vi "hostCommander_dualVStim.vi"() -> ()   [LabVIEW 2014]
uses:
  <vilib>/Platform/TimedLoop/XDataNode/timing_clust.ctl
  <vilib>/Platform/TimedLoop/XDataNode/nitl_modes.ctl
  <vilib>/Platform/TimedLoop/XDataNode/wakeup.ctl
  <vilib>/dex/Stream Element Allocation Mode.ctl
  <vilib>/platform/TimedLoop/XDataNode/XDataNode.xnode
  <resource>/objmgr/ni.dex.rc
  <vilib>/Platform/TimedLoop/XDataNode/XDNodeRunTimeDep.lvlib
  <vilib>/Analysis/NI_AALBase.lvlib
  <vilib>/Analysis/1siggen.llb/Riffle Array (I32).vi
panel:
  in  "allowCorrection 2":bool
  out "Tab Control":enum32{"Host Commander"}(tab)
  out "rightReward":dbl format="%.2f"
  out "leftReward":dbl format="%.2f"
  out "rightLick":dbl format="%.2f"
  out "leftLick":dbl format="%.2f"
  out "reward#":i32=500
  in  "tickRate":u32=1
  in  "displayLength":dbl=10.0
  out "CurTrial#":u16
  out "Digital Waveform Graph":digitalwaveform(graph)
  out "stateMissed":bool
  out "VSmissed":bool
  out "VSbusy":bool=TRUE caption="VS"
  out "stateBusy":bool=TRUE caption="State"
  in  "FileName":string="debug"
  in  "Save data":bool=TRUE
  in  "Tab Control _2":T1(tab)
  in  "trialKey":i32[](array[numeric])
  in  "left":dbl=0.5 format="%.2f"
  in  "right":dbl=0.5 format="%.2f"
  in  "Initializeation Screen":dbl
  in  "Repeat":dbl
  in  "Interleave":bool
  in  "Randominze":bool
  in  "Blank":bool
  in  "Timing":sgl[](array[numeric])=[0.1, 0.2, 0.4, 0.6, 0.8, 1.0]
  in  "Orientation":sgl[](array[numeric])=[0.1, 0.2, 0.4, 0.6, 0.8, 1.0]
  in  "TF":sgl[](array[numeric])=[0.1, 0.2, 0.4, 0.6, 0.8, 1.0]
  in  "VS type":string="LR_FullFiledGrating"
  in  "SF":sgl[](array[numeric])=[0.04, 0.08, 0.16, 0.32, 0.45]
  in  "rtFIFOsize":u32=50
  in  "rtFIFOtimeout":u32
  in  "rtFIFOdataPool":u32=20
  in  "stateMachineCycle_uS":i64=500
  in  "minDelay":i32
  in  "maxDelay":i32=2000000
  in  "autoAllowCorrection":bool
  in  "allowCorrection":bool=TRUE
  in  "autoDelay":bool
  in  "vsFilterPeriod_uS":i32=500 format="%#1.6f"
  in  "lickThreshold_V":fxp<+/-,16,5>=1.0 format="%#.4f"
  in  "vsThreshold_V":fxp<+/-,16,5>=2.0 format="%#.4f"
  in  "audioThreshold_V":fxp<+/-,16,5>=2.2998046875 format="%.4f"
  in  "audioFilterPeriod_uS":i32=500 format="%#1.6f"
  in  "audioOffState_V":fxp<+/-,16,5> format="%#.4f"
  in  "manualShock":bool
  in  "manualWaterRight":bool
  in  "manualWaterLeft":bool
  in  "lickReward":bool
  in  "allowPunish":bool
  in  "beh type":string="LeftRight"
  in  "toneReward":bool
  in  "rwdrefPeriod_uS":u32=1000000
  in  "rewardPeriod_uS":u32=3000000
  in  "waterOn_uS":u32=35000
  in  "timeout_uS":u32
  in  "shockOn_uS":u32
  in  "delay_uS":u32
  out "current state":u16(ring) items=["idle", "vs before", "vs", "vs after", "delay", "tone before", "tone", "tone after", "cycle end", "reward", "reward refractory", "punish", "punish refractory", "timeout", "exit"]
  out "case2":i32
  out "case1":i32
  in  "forceLeftTrial":bool
  in  "forceRightTrial":bool
  in  "forceCorrTrial":bool
  in  "autoCorrTrial":bool
  in  "autoTimeout":bool
  in  "autoStop":bool
  in  "autoStopAtReward#":i32=250
  in  "updateEveryTrial#":u16=10
  in  "maxTimeout":i32=8000000
  out "newStartTrial#":i32
  out "newStartReward#":i32
  out "contNoRewardAccum":i32
  out "contNoReward":i32
  out "contReward":i32
  out "curPerformance":dbl format="%.2f"
  out "overallPerformance":dbl format="%.2f"
  in  "waterPunish":bool
  in  "No VS":bool
  out "Error 1":string
  out "Error 2":string
  out "Originating IP":string="192.168.137.2"
  out "Incoming data":string="TrlDone 1.000 "
  out "stream counter":u32
  out "Is Connected":bool
  out "Available Elements for Writing":i32
  in  "stream writer buffer size":i32=500
  in  "IP_VS":string="192.168.137.3"
  in  "IP_RT":string="192.168.137.2"
  in  "port_remote":u16=9091
  in  "IP_host":string="192.168.137.1"
  in  "port_local":u16=9090
  in  "IP_broadcast":string="192.168.137.255"
  out "INFO":string="Stop 1.000 "
  out "stop - local":bool=TRUE
  in  "Notes":string="14-4"
  in  "Abort":bool caption="run-stop"
  in  "run-stop":bool
  out "dispTimeout":bool
  out "saveTimeout":bool
  out "CurTrial# (remote)":u16
  in  "totalTrial#":u16=600
  out "CurTime":i32
  in  "ITI_ms":dbl=2000.0
  out "CurTime (sec)":i32
  in  "FilePath":string="D:\\BehData\\"
  # "busy"
  # "missed"
  # "min"
  # "sec"
  # "trialProbability"
  # "Errors for debugging"
types:
  T1 = enum32{"Visual Stimuli", "State Machine", "Behavior", "Network", "Notes"}
  T2 = enum16{"open", "replace", "create", "open or create", "replace or create", "replace or create with confirmation"}
  T3 = enum16{"big-endian, network order", "native, host order", "little-endian"}
  T4 = typedef "XDNodeRunTimeDep.lvlib/timing_clust.ctl" = cluster{"Expected End [f-1]":u64, "Actual End [f-1]":u64, "Finished Late? [f-1]":bool, "Expected End [i-1]":u64, "Actual End [i-1]":u64, "Finished Late? [i-1]":bool, "Expected Start [i]":u64, "Actual Start [i]":u64, "Expected Start [f]":u64, "Actual Start [f]":u64, "Source Name":string, "Structure Name":string, "Period":i64, "Deadline":i64, "Offset":i64, "Start":i64, "Priority":i32, "Timeout":i32, "Mode":T5, "Wakeup Reason":T6, "Error":errorcluster, "Source Type":string, "Secondary Source Type":string, "Global End Time":u64, "Global Start Time":u64, "Frame Duration":u64, "Iteration Duration":u64, "Assigned CPU":i32, "I/O Scan Engine Mode":u32}
  T5 = typedef "XDNodeRunTimeDep.lvlib/nitl_modes.ctl" = enum32{"No Change", "Process missed periods, maintain original phase", "Discard missed periods, maintain original phase", "Process missed periods, ignore original phase", "Discard missed periods, ignore original phase"}
  T6 = typedef "XDNodeRunTimeDep.lvlib/wakeup.ctl" = enum32{"Normal", "Aborted", "Asynchronous wakeup", "Timing source error", "Timed loop error", "Timeout"}
  T7 = typedef "Stream Element Allocation Mode.ctl" = u32
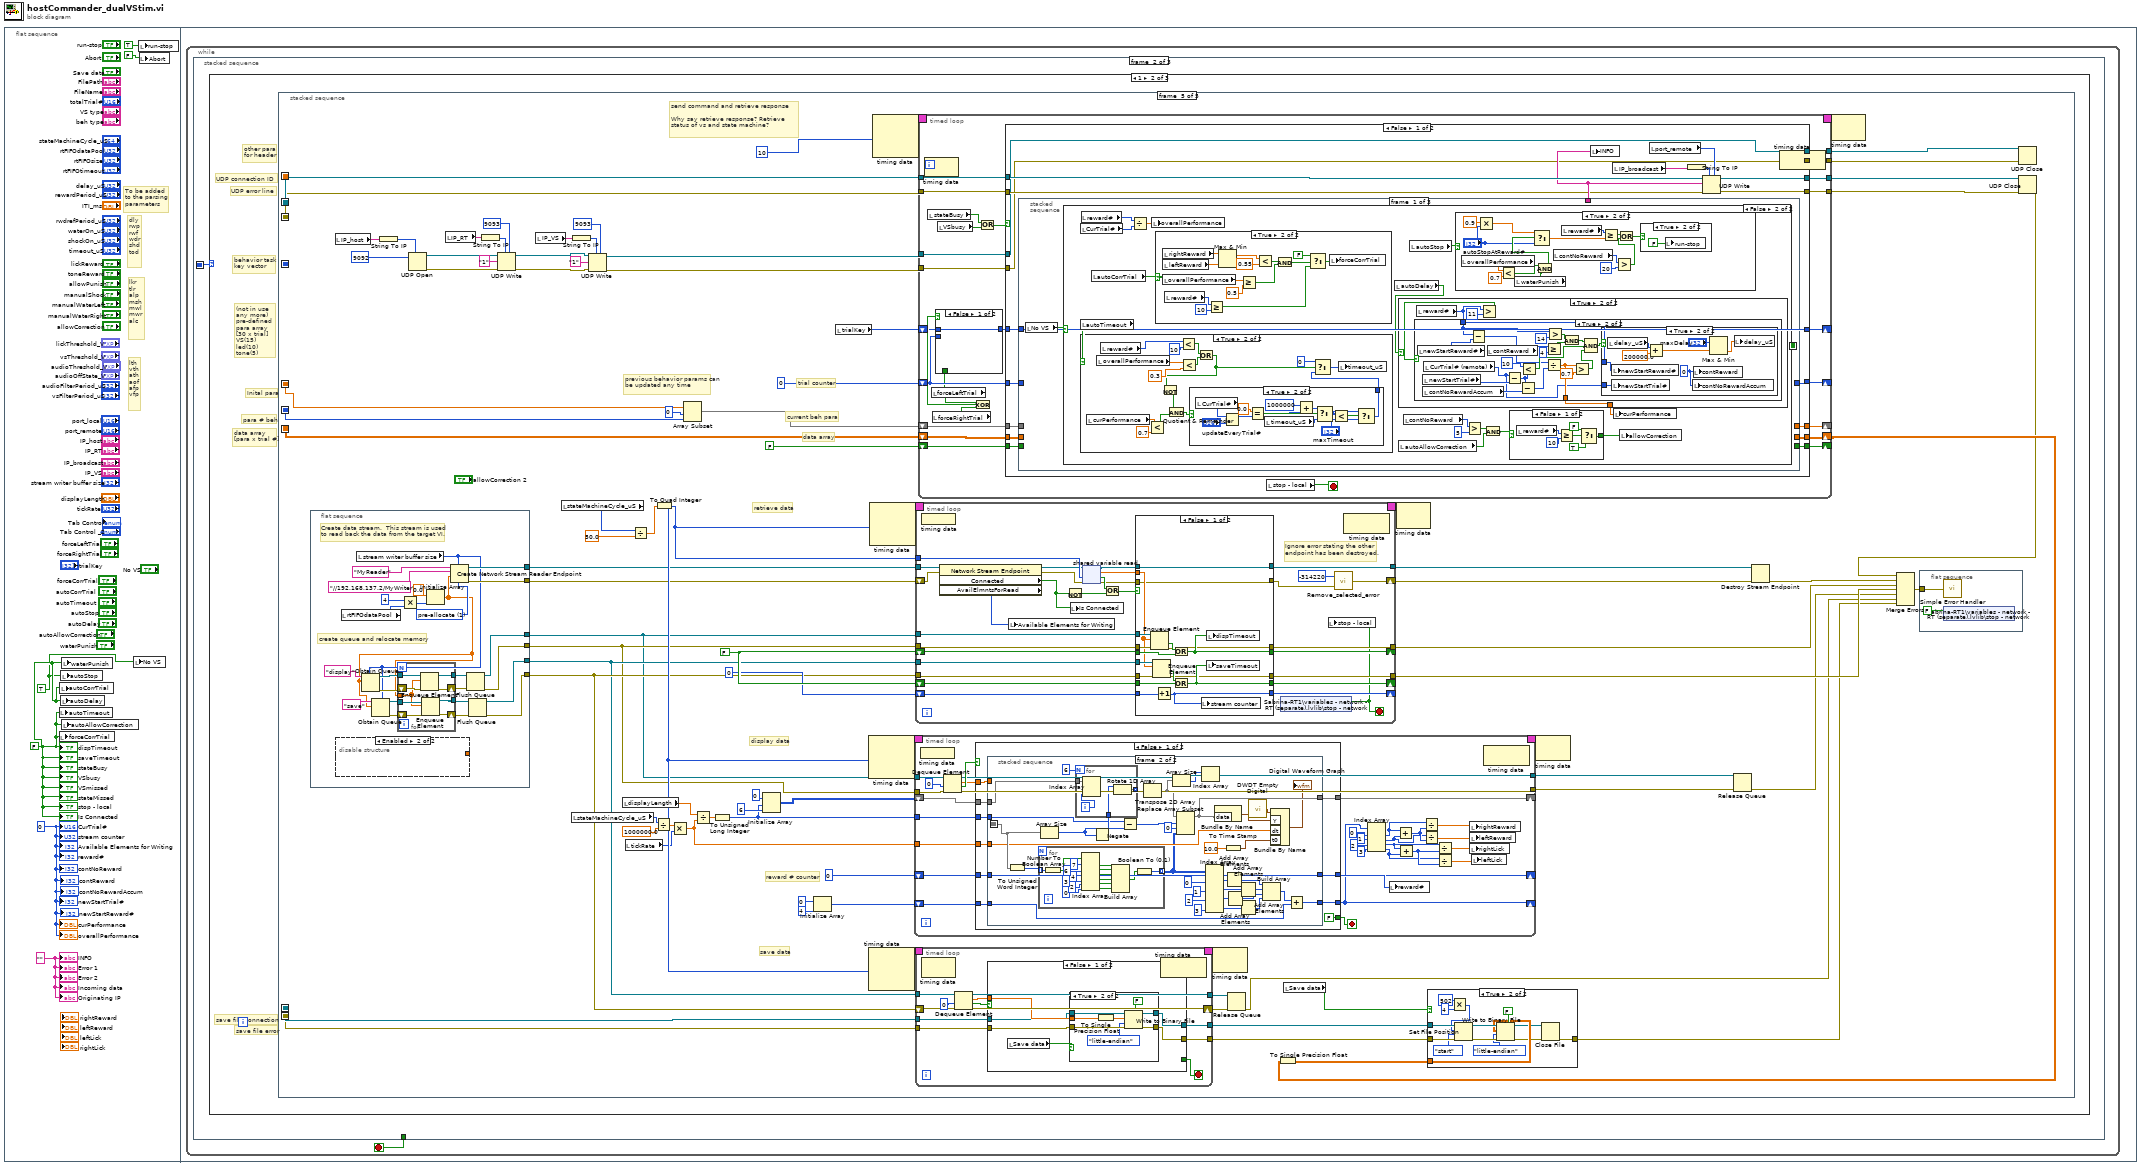
[diagram p0: block diagram]
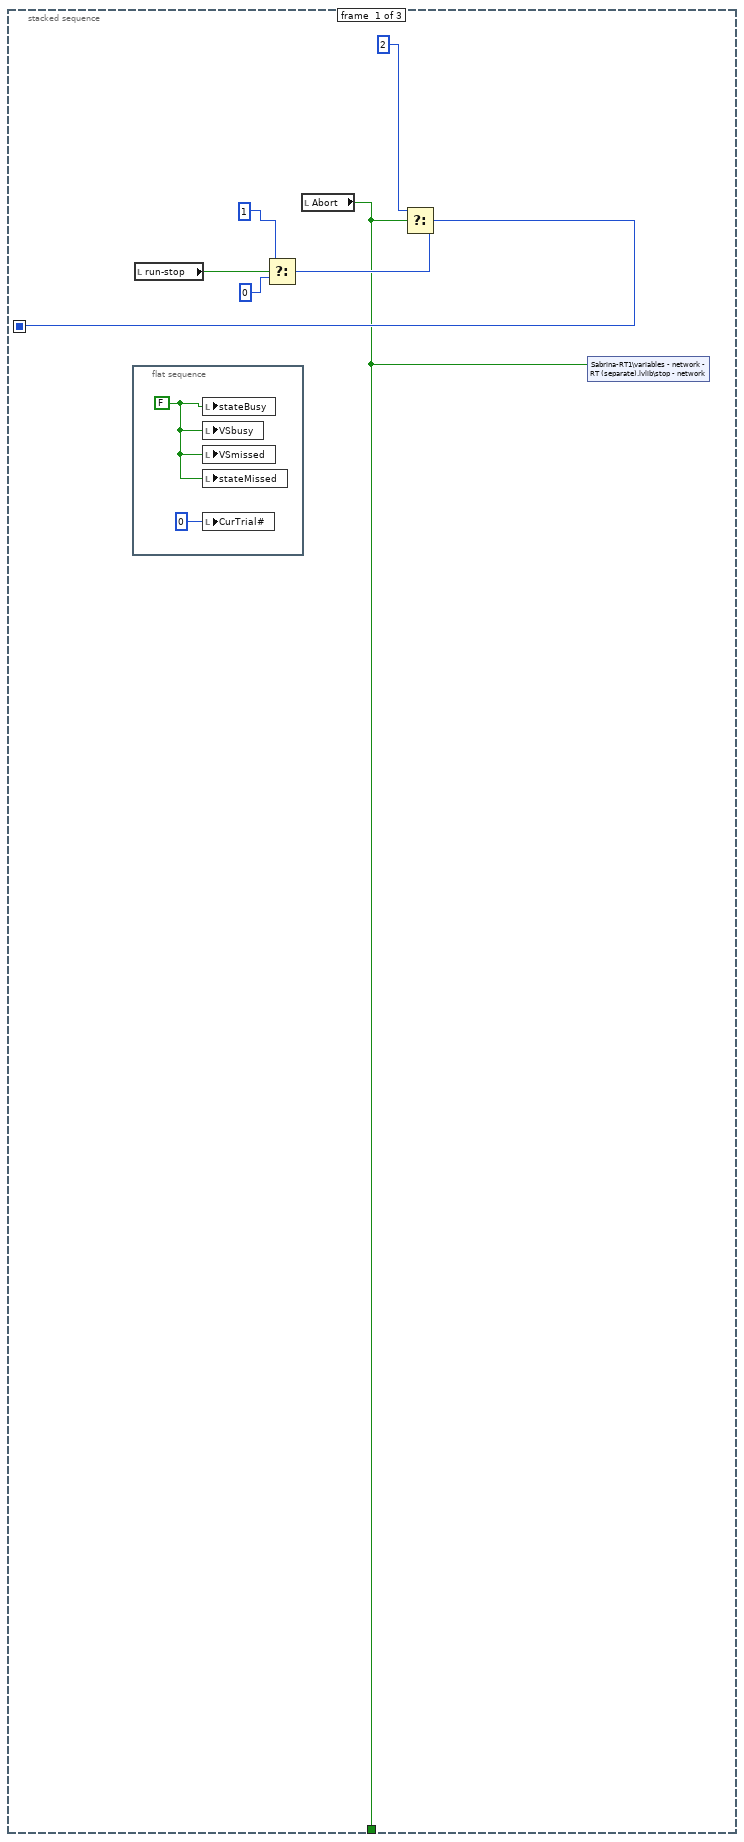
[diagram p2: hidden frame]
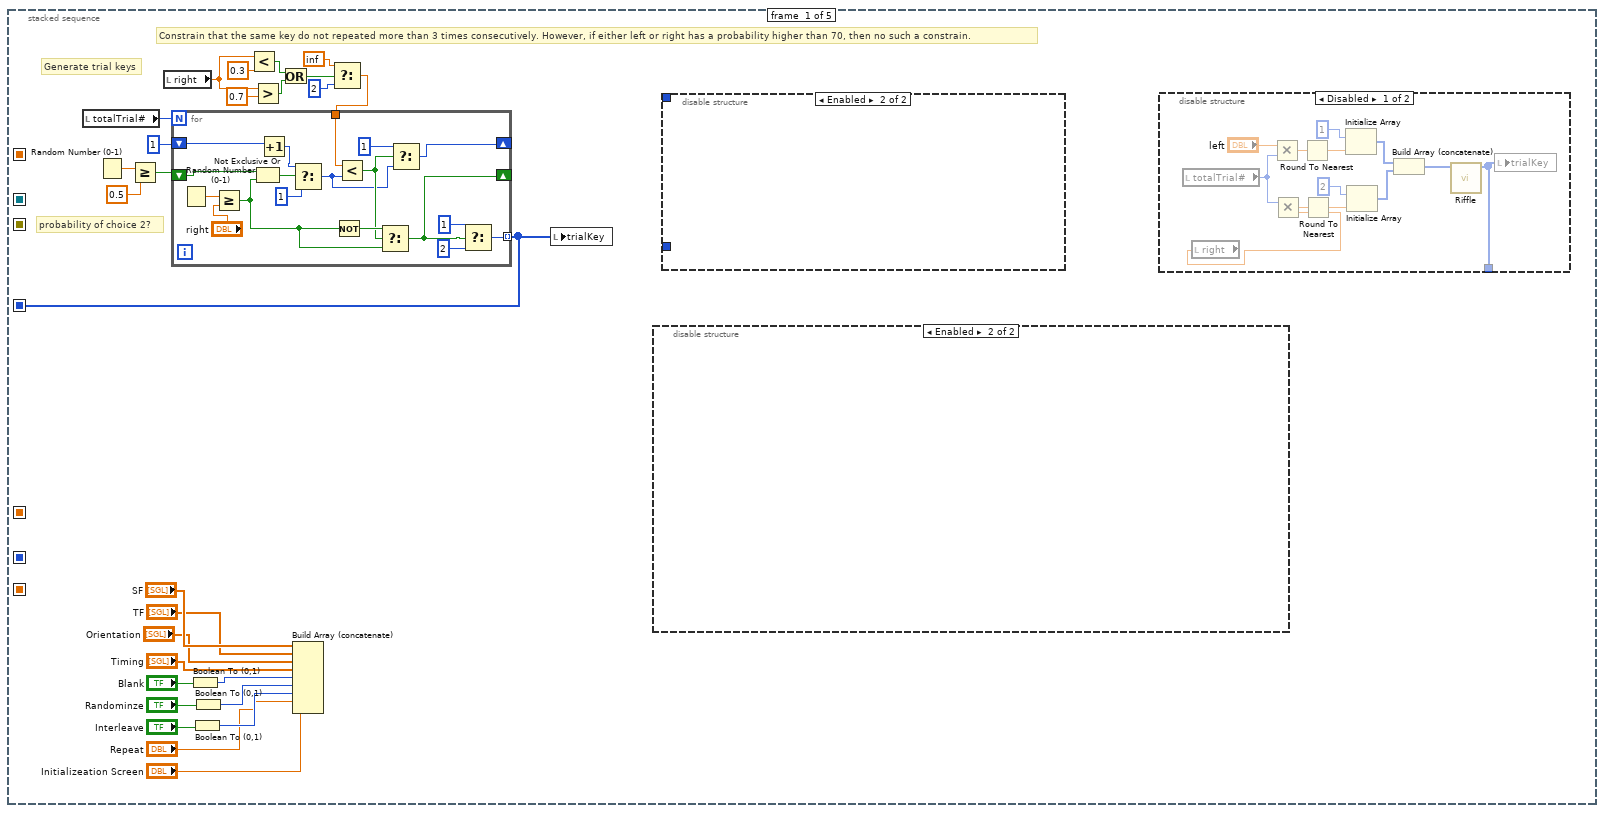
[diagram p4: hidden frame]
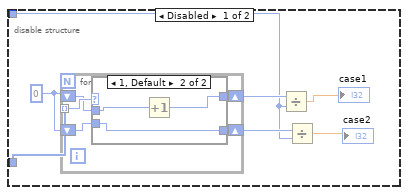
[diagram p5: hidden frame]
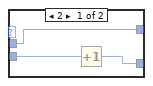
[diagram p6: hidden frame]
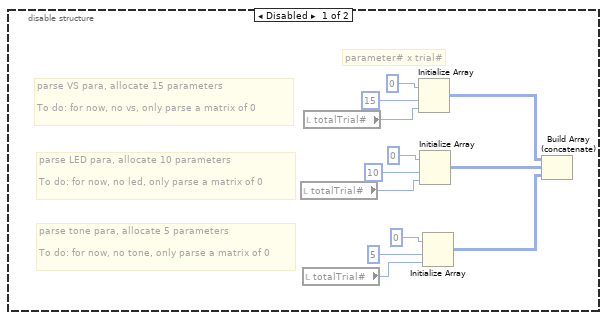
[diagram p8: hidden frame]
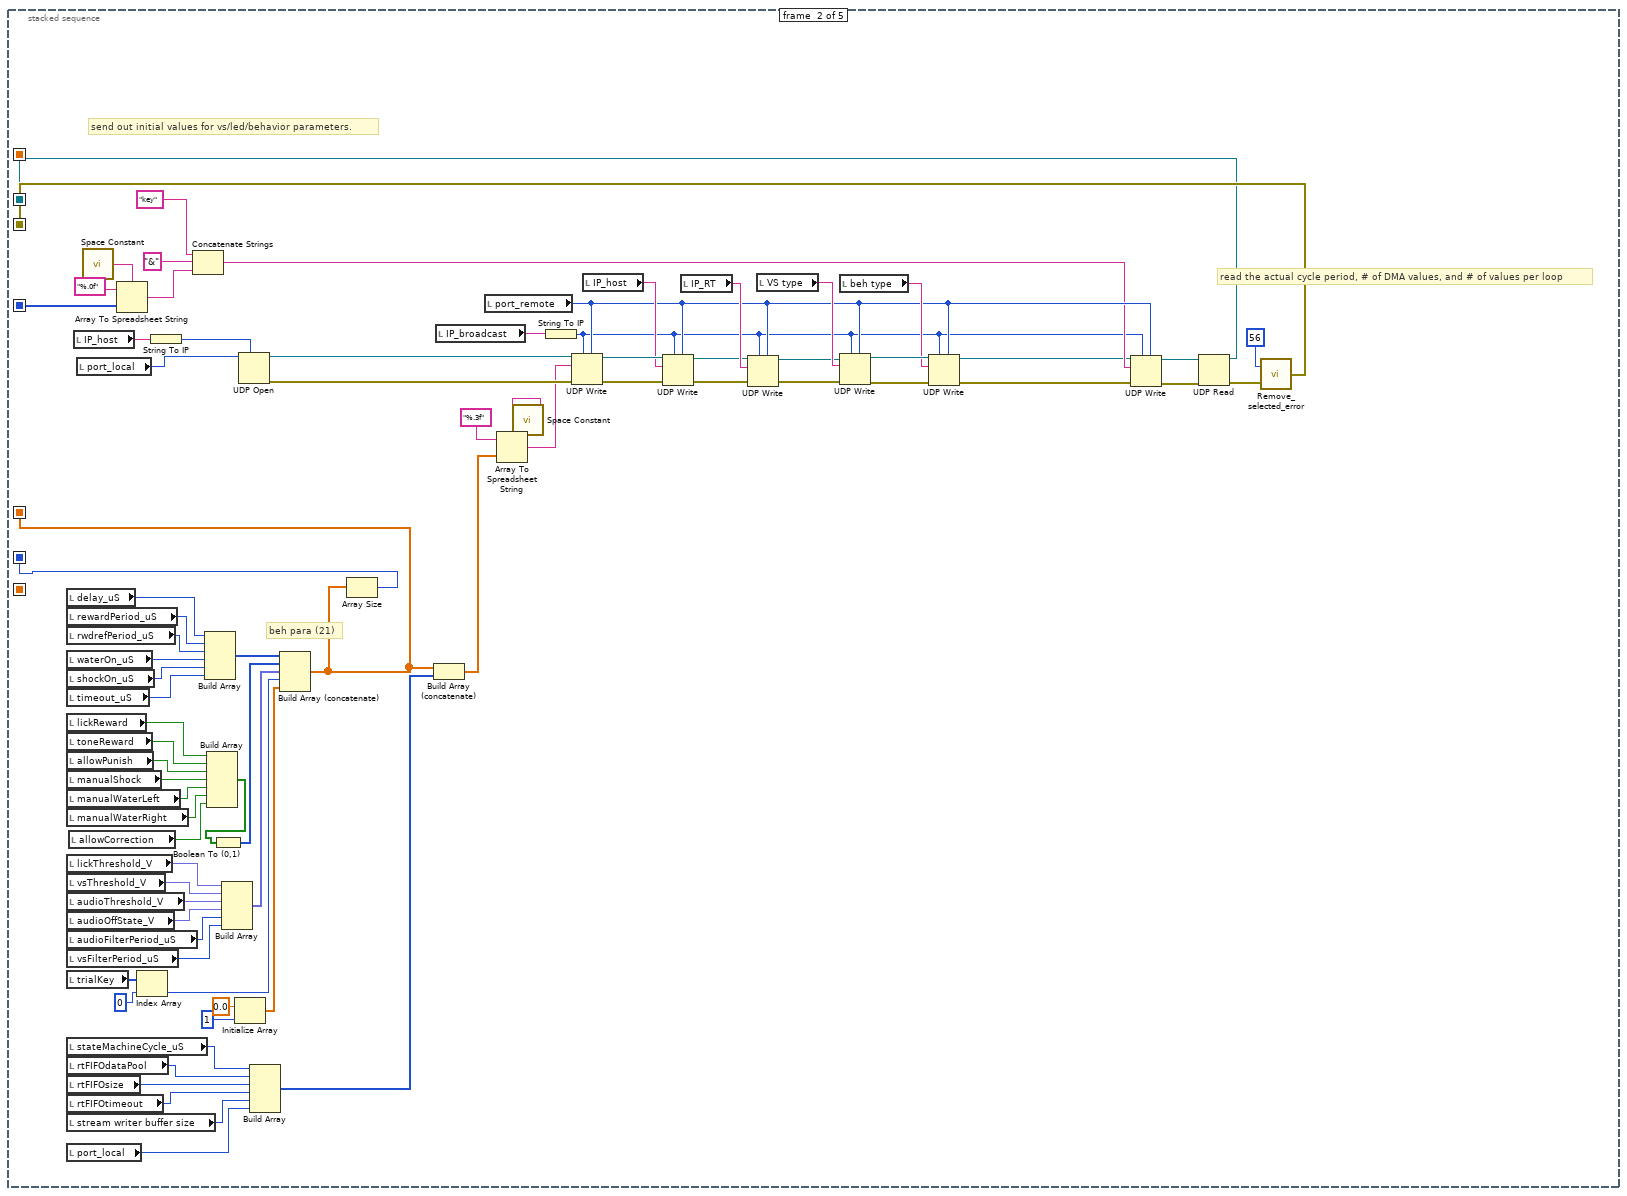
[diagram p9: hidden frame]
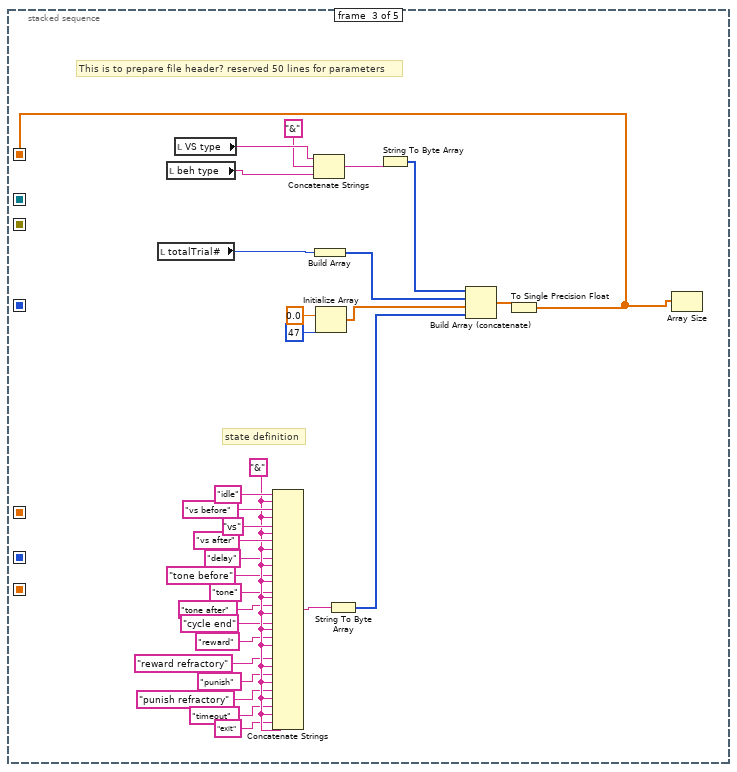
[diagram p10: hidden frame]
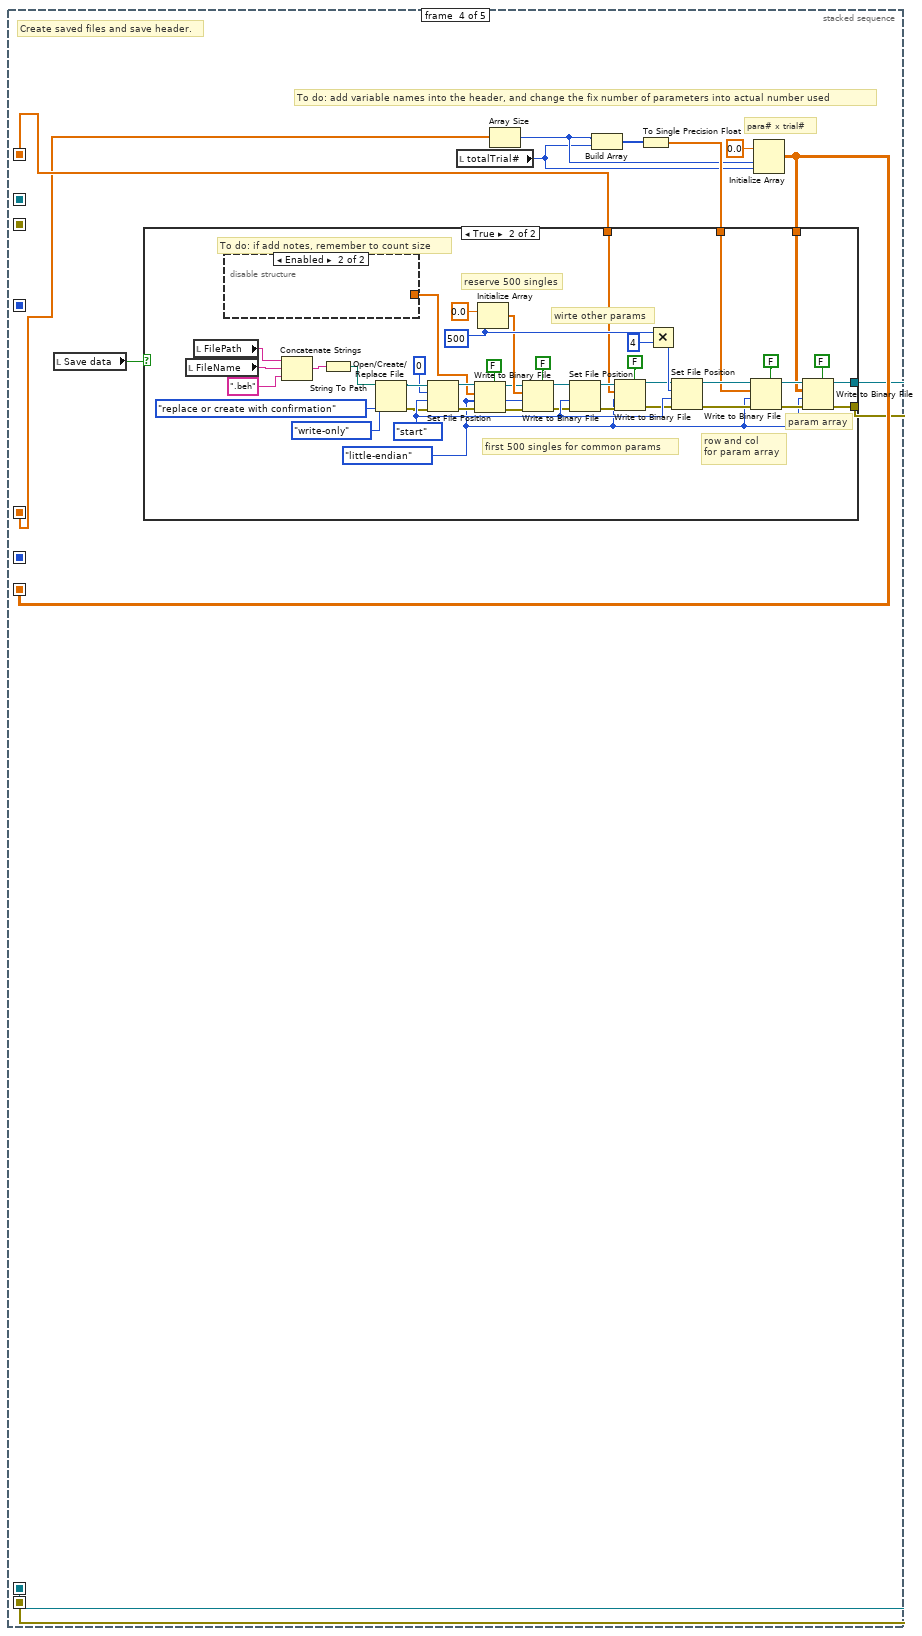
[diagram p11: hidden frame]
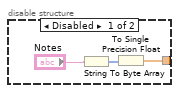
[diagram p13: hidden frame]
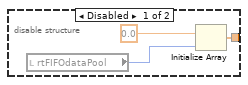
[diagram p14: hidden frame]
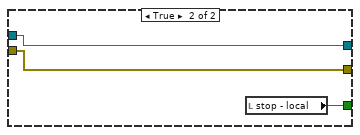
[diagram p16: hidden frame]
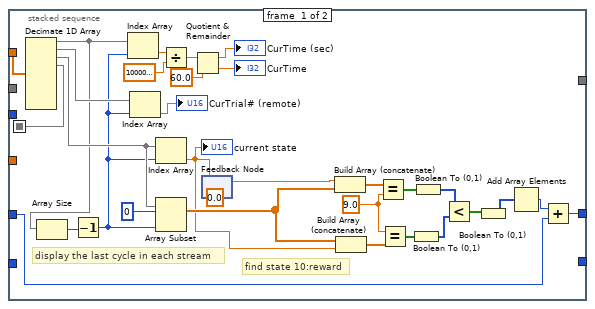
[diagram p17: hidden frame]
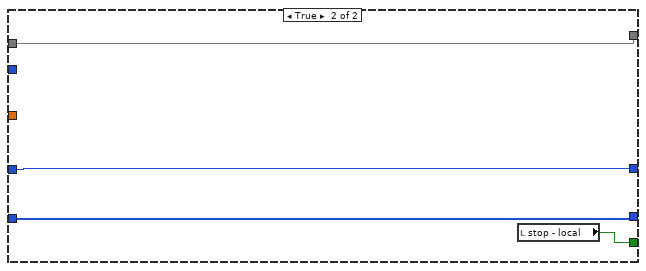
[diagram p18: hidden frame]
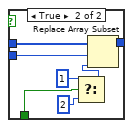
[diagram p20: hidden frame]
diagram:
  n1 = flat-sequence {
    frame #0 {
      w1 = TRUE
      w4 = ""
      w3 = 0
      w2 = FALSE
      # "To be added\nto the parsing\nparameters"
      # "lth\nvth\nath\naof\nafp\nvfp"
      # "dly\nrwp\nrwf\nwdr\nshd\ntod"
      # "lkr\ntlr\nalp\nmsh\nmwl\nmwr\nalc"
      n2 = local write "autoTimeout"(w2) -> ()
      n3 = local write "forceCorrTrial"(w2) -> ()
      n4 = local write "autoCorrTrial"(w2) -> ()
      n5 = local write "autoDelay"(w2) -> ()
      n6 = local write "autoStop"(w1) -> ()
      n7 = local write "waterPunish"(w2) -> ()
      n8 = local write "autoAllowCorrection"(w2) -> ()
      n9 = local write "No VS"(w1) -> ()
      n10 = local write "run-stop"(TRUE) -> ()
      n11 = local write "Abort"(FALSE) -> ()
      "dispTimeout" <- w2
      "saveTimeout" <- w2
      "stateBusy" <- w2
      "VSbusy" <- w2
      "VSmissed" <- w2
      "stateMissed" <- w2
      "CurTrial#" <- w3
      "stop - local" <- w2
      "INFO" <- w4
      "Error 2" <- w4
      "Error 1" <- w4
      "Available Elements for Writing" <- w3
      "Is Connected" <- w2
      "stream counter" <- w3
      "Incoming data" <- w4
      "Originating IP" <- w4
      "reward#" <- w3
      "contNoReward" <- w3
      "contReward" <- w3
      "contNoRewardAccum" <- w3
      "newStartTrial#" <- w3
      "newStartReward#" <- w3
      "curPerformance" <- w3
      "overallPerformance" <- w3
    }
    frame #1 {
      n12 = while {
        stop <- w7 stop-if-true
        n13 = stacked-sequence {
          seq-local: [w9 _ _] -> [_ w17 _]
          tunnel: [w8 _ _] -> w7
          frame #0 {
            n14 = flat-sequence {
              frame #0 {
                w16 = FALSE
                n15 = local write "stateBusy"(w16) -> ()
                n16 = local write "VSbusy"(w16) -> ()
                n17 = local write "VSmissed"(w16) -> ()
                n18 = local write "stateMissed"(w16) -> ()
                n19 = local write "CurTrial#"(0) -> ()
              }
            }
            n20 = local read "run-stop"() -> (w11:bool)
            n21 = Select(t=u8 1, s=w11, f=u8 0) -> (s? t:f=w10:u8)
            n22 = local read "Abort"() -> (w8:bool)
            n23 = Select(t=u8 2, s=w8, f=w10) -> (s? t:f=w9:u8)
            n24 = shared-variable "Sabrina-RT1\\variables - network - RT (separate).lvlib\\stop - network"(w8) -> ()  [unwired: 1 in, 1 out]
          }
          frame #1 {
            n25 = case shown="1" w17 {
              frame 0, Default {
              }
              frame 1 {
                # "behavior task\nkey vector"
                # "para # beh"
                # "save file error"
                # "save file connection"
                # "data array\n[para x trial #]"
                # "other para\nfor header"
                # "UDP error line"
                # "UDP connection ID"
                # "Inital para"
                # "(not in use any more) pre-defined \npara array\n[30 x trial]\nVS(15)\nled(10)\ntone(5)"
                n26 = stacked-sequence {
                  seq-local: [_ w166 _ _ _] -> [_ _ _ _ w342]
                  seq-local: [_ w165 _ _ _] -> [_ _ _ _ w343]
                  seq-local: [_ w125 _ _ _] -> [_ _ _ w215 w291]
                  seq-local: [w18 _ _ _ _] -> [_ w121 _ _ _]
                  seq-local: [_ _ w183 _ _] -> [_ _ _ w219 _]
                  seq-local: [_ _ _ w218 _] -> [_ _ _ _ w336]
                  seq-local: [_ _ _ w217 _] -> [_ _ _ _ w316]
                  seq-local: [_ _ _ w216 _] -> [_ _ _ _ w317]
                  seq-local: [_ w134 _ _ _] -> [_ _ _ _ w297]
                  frame #0 {
                    # "probability of choice 2?"
                    # "Constrain that the same key do not repeated more than 3 times consecutively. However, if either left or right has a probability higher than 70, then no such a constrain."
                    # "Generate trial keys"
                    n27 = local read "totalTrial#"() -> (w19:u16)
                    n28 = Random Number (0-1)() -> (number: 0 to 1=w32:dbl)
                    n29 = Greater Or Equal?(x=w32, y=0.5) -> (x >= y?=w30:bool)
                    n30 = local read "right"() -> (w26:dbl)
                    n31 = Boolean To (0,1)(Boolean="Blank") -> (0, 1=w39:i16)
                    n32 = Boolean To (0,1)(Boolean="Interleave") -> (0, 1=w34:i16)
                    n33 = Boolean To (0,1)(Boolean="Randominze") -> (0, 1=w38:i16)
                    n34 = Less?(x=w26, y=0.3) -> (x < y?=w23:bool)
                    n35 = Greater?(x=w26, y=0.7) -> (0:w22:bool)
                    n36 = Or(x=w23, y=w22) -> (x .or. y?=w21:bool)
                    n37 = Build Array (concatenate)("SF", "TF", "Orientation", "Timing", w39, w38, w34, "Repeat", "Initializeation Screen") -> ()  [unwired: 1 out]
                    n38 = Select(t=inf, s=w21, f=2) -> (s? t:f=w20:dbl)
                    n39 = for {
                      N: w19 -> [_]
                      shift-right: [w79] -> _
                      shift-left: w30 -> [w92]
                      shift-right: [w77] -> _
                      shift-left: 1 -> [w90]
                      tunnel: w20 -> [w80]
                      tunnel: [w78] -> w18 mode=indexing
                      n40 = Random Number (0-1)() -> (number: 0 to 1=w93:dbl)
                      n41 = Greater Or Equal?(x=w93, y="right") -> (x >= y?=w83:bool)
                      n42 = Not Exclusive Or(1:w83, 2:w92) -> (0:w91:bool)
                      n43 = Increment(x=w90) -> (x+1=w87:i32)
                      n44 = Select(t=w87, s=w91, f=1) -> (s? t:f=w81:i32)
                      n45 = Not(x=w83) -> (.not. x?=w84:bool)
                      n46 = Less?(x=w80, y=w81) -> (x < y?=w82:bool)
                      n47 = Select(t=w84, s=w82, f=w83) -> (s? t:f=w79:bool)
                      n48 = Select(t=1, s=w82, f=w81) -> (s? t:f=w77:i32)
                      n49 = Select(t=1, s=w79, f=2) -> (s? t:f=w78:i32)
                    }
                    n50 = local write "trialKey"(w18) -> ()
                    n51 = disable-structure shown="Enabled" {
                      frame Disabled {
                        # "parameter# x trial#"
                        # "parse tone para, allocate 5 parameters \n\nTo do: for now, no tone, only parse a matrix of 0"
                        # "parse LED para, allocate 10 parameters \n\nTo do: for now, no led, only parse a matrix of 0"
                        # "parse VS para, allocate 15 parameters \n\nTo do: for now, no vs, only parse a matrix of 0"
                        n52 = local read "totalTrial#"() -> (w99:u16)
                        n53 = local read "totalTrial#"() -> (w98:u16)
                        n54 = local read "totalTrial#"() -> (w100:u16)
                        n55 = Initialize Array(0, 15, w100) -> (w103:i32[][])
                        n56 = Initialize Array(0, 10, w99) -> (w102:i32[][])
                        n57 = Initialize Array(0, 5, w98) -> (w101:i32[][])
                        n58 = Build Array (concatenate)(w103, w102, w101) -> ()  [unwired: 1 out]
                      }
                      frame Enabled {
                      }
                    }
                    n59 = disable-structure shown="Enabled" {
                      disable-tunnel: _ -> [w51 _]
                      disable-tunnel: _ -> [w45 _]
                      frame Disabled {
                        w50 = 0
                        n60 = for {
                          tunnel: w51 -> [w56] mode=indexing
                          shift-right: [w54] -> w47
                          shift-left: w50 -> [w55]
                          shift-right: [w52] -> w49
                          shift-left: w50 -> [w53]
                          n61 = case shown="1, Default" w56 {
                            tunnel: w55 -> [w59 w60]
                            tunnel: [w58 w60] -> w54
                            tunnel: w53 -> [w57 w62]
                            tunnel: [w57 w61] -> w52
                            frame 2 {
                              n62 = Increment(x=w59) -> (x+1=w58:i32)
                            }
                            frame 1, Default {
                              n63 = Increment(x=w62) -> (x+1=w61:i32)
                            }
                          }
                        }
                        n64 = Divide(x=w49, y=w45) -> (x/y=→"case1":dbl)
                        n65 = Divide(x=w47, y=w45) -> (x/y=→"case2":dbl)
                      }
                      frame Enabled {
                      }
                    }
                    n66 = disable-structure shown="Disabled" {
                      disable-tunnel: [w64 _] -> _
                      frame Disabled {
                        n67 = local read "totalTrial#"() -> (w68:u16)
                        n68 = local read "right"() -> (w63:dbl)
                        n69 = Multiply(x="left", y=w68) -> (x*y=w74:dbl)
                        n70 = Multiply(x=w68, y=w63) -> (x*y=w69:dbl)
                        n71 = Round To Nearest(number=w74) -> (nearest integer value=w72:dbl)
                        n72 = Round To Nearest(number=w69) -> (nearest integer value=w71:dbl)
                        n73 = Initialize Array(1, w72) -> (w67:i32[])
                        n74 = Initialize Array(2, w71) -> (w66:i32[])
                        n75 = Build Array (concatenate)(w67, w66) -> (w65:i32[])
                        n76 = call-poly <vilib>:"Riffle.vi"("X"=w65) -> ("Riffled {X}"=w64:i32[])  [unwired: 8 in, 2 out]
                        n77 = local write "trialKey"(w64) -> ()
                      }
                      frame Enabled {
                      }
                    }
                  }
                  frame #1 {
                    # "beh para (21)"
                    # "read the actual cycle period, # of DMA values, and # of values per loop"
                    # "send out initial values for vs/led/behavior parameters."
                    n78 = local read "delay_uS"() -> (w162:u32)
                    n79 = local read "rewardPeriod_uS"() -> (w161:u32)
                    n80 = local read "rwdrefPeriod_uS"() -> (w160:u32)
                    n81 = local read "waterOn_uS"() -> (w159:u32)
                    n82 = local read "shockOn_uS"() -> (w158:u32)
                    n83 = local read "timeout_uS"() -> (w157:u32)
                    n84 = local read "lickReward"() -> (w156:bool)
                    n85 = local read "toneReward"() -> (w155:bool)
                    n86 = local read "allowPunish"() -> (w154:bool)
                    n87 = local read "manualShock"() -> (w153:bool)
                    n88 = local read "manualWaterLeft"() -> (w152:bool)
                    n89 = local read "manualWaterRight"() -> (w151:bool)
                    n90 = local read "lickThreshold_V"() -> (w150:fxp<+/-,16,5>)
                    n91 = local read "vsThreshold_V"() -> (w149:fxp<+/-,16,5>)
                    n92 = local read "audioThreshold_V"() -> (w148:fxp<+/-,16,5>)
                    n93 = local read "audioOffState_V"() -> (w145:fxp<+/-,16,5>)
                    n94 = local read "audioFilterPeriod_uS"() -> (w147:i32)
                    n95 = local read "vsFilterPeriod_uS"() -> (w146:i32)
                    n96 = local read "trialKey"() -> (w110:i32[])
                    n97 = local read "stateMachineCycle_uS"() -> (w144:i64)
                    n98 = local read "rtFIFOdataPool"() -> (w142:u32)
                    n99 = local read "rtFIFOsize"() -> (w141:u32)
                    n100 = local read "rtFIFOtimeout"() -> (w143:u32)
                    n101 = local read "stream writer buffer size"() -> (w140:i32)
                    n102 = local read "port_local"() -> (w133:u16)
                    n103 = local read "allowCorrection"() -> (w106:bool)
                    n104 = local read "IP_host"() -> (w179:string)
                    n105 = local read "port_local"() -> (w178:u16)
                    n106 = call <vilib>:"Space Constant.vi"() -> ("String"=w115:string)
                    n107 = Array To Spreadsheet String ("beh para")(delimiter (Tab)=w115, array=w121, 3:"%.0f" ("format string")) -> (spreadsheet string=w117:string)
                    n108 = Index Array(array=w110, index=0) -> (element=w107:i32)
                    n109 = String To IP(1:w179) -> (0:w111:u32)
                    n110 = Concatenate Strings("key", "&", w117) -> (w116:string)
                    n111 = Build Array(w162, w161, w160, w159, w158, w157) -> (w139:u32[])
                    n112 = Build Array(w156, w155, w154, w153, w152, w151, w106) -> (w127:bool[])
                    n113 = Boolean To (0,1)(Boolean=w127) -> (0, 1=w126:i16[])
                    n114 = Build Array(w150, w149, w148, w145, w147, w146) -> (w138:fxp<+/-,43,32>[])
                    n115 = Initialize Array(sgl 0.0, 1) -> (w108:sgl[])
                    n116 = UDP Open(7:w111, 11:w178) -> (port=w176:refnum<k16>, 0:w177:errorcluster)  [unwired: 3 in, 1 out]
                    n117 = Build Array(w144, w142, w141, w143, w140, w133) -> (w137:i64[])
                    n118 = Build Array (concatenate)(w139, w126, w138, w107, w108) -> (w125:sgl[])
                    n119 = Array Size(array=w125) -> (size(s)=w134:i32)
                    n120 = Build Array (concatenate)(w125, w137) -> (w167:sgl[])
                    n121 = local read "IP_broadcast"() -> (w180:string)
                    n122 = local read "port_remote"() -> (w118:u16)
                    n123 = call <vilib>:"Space Constant.vi"() -> ("String"=w169:string)
                    n124 = Array To Spreadsheet String ("beh para")(delimiter (Tab)=w169, array=w167, 3:"%.3f" ("format string")) -> (spreadsheet string=w168:string)
                    n125 = String To IP(1:w180) -> (0:w112:u32)
                    n126 = UDP Write(address=w112, port or service name=w118, connection ID=w176, data in=w168, 8:w177) -> (error out=w175:errorcluster, 3:w132:refnum<k16>)  [unwired: 1 in]
                    n127 = local read "IP_host"() -> (w131:string)
                    n128 = UDP Write(address=w112, port or service name=w118, connection ID=w132, data in=w131) -> (3:w129:refnum<k16>)  [unwired: 2 in, 1 out]
                    n129 = local read "IP_RT"() -> (w130:string)
                    n130 = UDP Write(address=w112, port or service name=w118, connection ID=w129, data in=w130) -> (3:w128:refnum<k16>)  [unwired: 2 in, 1 out]
                    n131 = local read "VS type"() -> (w174:string)
                    n132 = local read "beh type"() -> (w171:string)
                    n133 = UDP Write(address=w112, port or service name=w118, connection ID=w128, data in=w174, 8:w175) -> (error out=w173:errorcluster, 3:w172:refnum<k16>)  [unwired: 1 in]
                    n134 = UDP Write(address=w112, port or service name=w118, connection ID=w172, data in=w171, 8:w173) -> (error out=w113:errorcluster, 3:w114:refnum<k16>)  [unwired: 1 in]
                    n135 = UDP Write(address=w112, port or service name=w118, connection ID=w114, data in=w116, 8:w113) -> (error out=w124:errorcluster, 3:w123:refnum<k16>)  [unwired: 1 in]
                    n136 = UDP Read(connection ID=w123, 8:w124) -> (error out=w164:errorcluster, 3:w165:refnum<k16>)  [unwired: 2 in, 3 out]
                    n137 = call "Remove_selected_error.vi"("error in (no error)"=w164, "errorCode"=56) -> ("error out"=w166:errorcluster)
                  }
                  frame #2 {
                    w195 = "&" ("string")
                    # "state definition"
                    # "This is to prepare file header? reserved 50 lines for parameters"
                    n138 = local read "totalTrial#"() -> (w203:u16)
                    n139 = local read "beh type"() -> (w181:string)
                    n140 = local read "VS type"() -> (w198:string)
                    n141 = Concatenate Strings("idle", w195, "vs before", w195, "vs", w195, "vs after", w195, "delay", w195, "tone before", w195, "tone", w195, "tone after", w195, "cycle end", w195, "reward", w195, "reward refractory", w195, "punish", w195, "punish refractory", w195, "timeout", w195, "exit", w195) -> (w208:string)
                    n142 = Concatenate Strings(w198, "&" ("string"), w181) -> (w197:string)
                    n143 = Build Array(w203) -> (w202:u16[])
                    n144 = Initialize Array(sgl 0.0 ("element"), 47 ("dimension size")) -> (w201:sgl[])
                    n145 = String To Byte Array(string=w208) -> (unsigned byte array=w200:u8[])
                    n146 = String To Byte Array(string=w197) -> (unsigned byte array=w196:u8[])
                    n147 = Build Array (concatenate)(w196, w202, w201, w200) -> (w199:sgl[])
                    n148 = To Single Precision Float(number=w199) -> (single precision float=w183:sgl[])
                    n149 = Array Size(array=w183) -> ()  [unwired: 1 out]
                  }
                  frame #3 {
                    # "To do: add variable names into the header, and change the fix number of parameters into actual number used"
                    # "para# x trial#"
                    # "Create saved files and save header."
                    n150 = local read "Save data"() -> (w221:bool)
                    n151 = local read "totalTrial#"() -> (w211:u16)
                    n152 = Array Size(array=w215) -> (size(s)=w212:i32)
                    n153 = Build Array(w212, w211) -> (w214:i32[])
                    n154 = To Single Precision Float(number=w214) -> (single precision float=w213:sgl[])
                    n155 = Initialize Array(sgl 0.0 ("element"), w212, w211) -> (w218:sgl[][])
                    n156 = case shown="True" w221 {
                      tunnel: w213 -> [_ w238]
                      tunnel: w219 -> [_ w222]
                      tunnel: w218 -> [_ w237]
                      tunnel: [_ w235] -> w216
                      tunnel: [_ w236] -> w217
                      frame False {
                      }
                      frame True {
                        w256 = 500 ("dimension size")
                        w229 = T3."little-endian" ("byte order (0:big-endian, network order)")
                        w257 = enum16{"start", "end", "current"}."start" ("from (0:start)")
                        # "To do: if add notes, remember to count size"
                        # "param array"
                        # "row and col\nfor param array"
                        # "first 500 singles for common params"
                        # "reserve 500 singles"
                        # "wirte other params"
                        n157 = local read "FileName"() -> (w224:string)
                        n158 = local read "FilePath"() -> (w227:string)
                        n159 = disable-structure shown="Enabled" {
                          disable-tunnel: [w264 _] -> w228
                          frame Disabled {
                            n160 = String To Byte Array(string="Notes") -> (unsigned byte array=w265:u8[])
                            n161 = To Single Precision Float(number=w265) -> (single precision float=w264:sgl[])
                          }
                          frame Enabled {
                          }
                        }
                        n162 = Concatenate Strings(w227, w224, ".beh" ("string")) -> (w226:string)
                        n163 = String To Path(string=w226) -> (path=w225:path)
                        n164 = Open/Create/Replace File(file path (use dialog)=w225, operation (0:open)=T2."replace or create with confirmation", access (0:read/write)=enum16{"read/write", "read-only", "write-only"}."write-only") -> (refnum out=w242:refnum<file>, error out=w243:errorcluster)  [unwired: 3 in, 1 out]
                        n165 = Set File Position(offset (in bytes) (0)=i64 0, refnum=w242, from (0:start)=w257, error in=w243) -> (refnum out=w233:refnum<file>, error out=w231:errorcluster)
                        n166 = Write to Binary File(file (use dialog)=w233, data=w228, error in=w231, 5:FALSE ("prepend array or string size? (T)"), 9:w229) -> (refnum out=w232:refnum<file>, error out=w230:errorcluster)  [unwired: 1 in, 1 out]
                        n167 = Initialize Array(sgl 0.0 ("element"), w256) -> (w246:sgl[])
                        n168 = Write to Binary File(file (use dialog)=w232, data=w246, error in=w230, 5:FALSE ("prepend array or string size? (T)"), 9:w229) -> (refnum out=w248:refnum<file>, error out=w249:errorcluster)  [unwired: 1 in, 1 out]
                        n169 = Set File Position(refnum=w248, from (0:start)=w257, error in=w249) -> (refnum out=w250:refnum<file>, error out=w251:errorcluster)  [unwired: 1 in]
                        n170 = Write to Binary File(file (use dialog)=w250, data=w222, error in=w251, 5:FALSE ("prepend array or string size? (T)"), 9:w229) -> (refnum out=w252:refnum<file>, error out=w253:errorcluster)  [unwired: 1 in, 1 out]
                        n171 = Multiply(x=w256, y=4) -> (x*y=w254:i32)
                        n172 = Set File Position(offset (in bytes) (0)=w254, refnum=w252, from (0:start)=w257, error in=w253) -> (refnum out=w259:refnum<file>, error out=w260:errorcluster)
                        n173 = Write to Binary File(file (use dialog)=w259, data=w238, error in=w260, 5:FALSE ("prepend array or string size? (T)"), 9:w229) -> (refnum out=w261:refnum<file>, error out=w262:errorcluster)  [unwired: 1 in, 1 out]
                        n174 = Write to Binary File(file (use dialog)=w261, data=w237, error in=w262, 5:FALSE ("prepend array or string size? (T)"), 9:w229) -> (refnum out=w235:refnum<file>, error out=w236:errorcluster)  [unwired: 1 in, 1 out]
                      }
                    }
                  }
                  frame #4 {
                    w348 = FALSE
                    # "reward # counter"
                    # "save data"
                    # "data array"
                    # "current beh para"
                    # "trial counter"
                    # "previous behavior params can be updated any time"
                    # "display data"
                    # "retrieve data"
                    # "send command and retrieve response\n\nWhy say retrieve response? Retrieve\nstatus of vs and state machine?"
                    n175 = flat-sequence {
                      tunnel: [w375] -> w303
                      tunnel: [w374] -> w302
                      tunnel: [w363] -> w301
                      tunnel: [w362] -> w300
                      tunnel: [w361] -> w299
                      tunnel: [w360] -> w298
                      frame #0 {
                        w377 = T7 1 items=["allocate as needed", "pre-allocate"] ("element allocation mode")
                        # "create queue and relocate memory"
                        # "Create data stream.  This stream is used\nto read back the data from the target VI."
                        n176 = disable-structure shown="Enabled" {
                          disable-tunnel: [w380 _] -> _
                          frame Disabled {
                            n177 = local read "rtFIFOdataPool"() -> (w381:u32)
                            n178 = Initialize Array(sgl 0.0, w381) -> (w380:sgl[])
                          }
                          frame Enabled {
                          }
                        }
                        n179 = local read "rtFIFOdataPool"() -> (w356:u32)
                        n180 = local read "stream writer buffer size"() -> (w359:i32)
                        n181 = Multiply(x=4, y=w356) -> (x*y=w355:u32)
                        n182 = Initialize Array(sgl 0.0, w355) -> (w358:sgl[])
                        n183 = Obtain Queue(max queue size (-1, unlimited)=w359, name (unnamed)="display", element data type=w358) -> (queue out=w366:refnum<queue>, error out=w367:errorcluster)  [unwired: 2 in, 1 out]
                        n184 = Obtain Queue(max queue size (-1, unlimited)=w359, name (unnamed)="save", element data type=w358) -> (queue out=w368:refnum<queue>, error out=w369:errorcluster)  [unwired: 2 in, 1 out]
                        n185 = for {
                          N: w359 -> [_]
                          tunnel: w366 -> [w391]
                          tunnel: [w390] -> w372
                          shift-right: [w388] -> w373
                          shift-left: w367 -> [w389]
                          shift-right: [w384] -> w371
                          shift-left: w369 -> [w385]
                          tunnel: w368 -> [w387]
                          tunnel: [w386] -> w370
                          tunnel: w358 -> [w383]
                          n186 = Enqueue Element(queue=w391, element=w383, error in (no error)=w389) -> (queue out=w390:refnum<queue>, error out=w388:errorcluster)  [unwired: 1 in, 1 out]
                          n187 = Enqueue Element(queue=w387, element=w383, error in (no error)=w385) -> (queue out=w386:refnum<queue>, error out=w384:errorcluster)  [unwired: 1 in, 1 out]
                        }
                        n188 = Create Network Stream Reader Endpoint(6:w377, 7:w359, 9:w358, 10:"//192.168.137.2/MyWriter" ("reader name"), 11:"MyReader" ("reader name")) -> (0:w375:errorcluster, 3:w374:refnum<k21>)  [unwired: 2 in]
                        n189 = Flush Queue(queue=w372, error in (no error)=w373) -> (queue out=w360:refnum<queue>, error out=w361:errorcluster)  [unwired: 1 out]
                        n190 = Flush Queue(queue=w370, error in (no error)=w371) -> (queue out=w362:refnum<queue>, error out=w363:errorcluster)  [unwired: 1 out]
                      }
                    }
                    n191 = local read "IP_host"() -> (w286:string)
                    n192 = String To IP(1:w286) -> (0:w285:u32)
                    n193 = UDP Open(7:w285, 11:9092) -> (port=w280:refnum<k16>, 0:w281:errorcluster)  [unwired: 3 in, 1 out]
                    n194 = local read "IP_RT"() -> (w279:string)
                    n195 = String To IP(1:w279) -> (0:w278:u32)
                    n196 = UDP Write(address=w278, port or service name=u16 9093, connection ID=w280, data in="1", 8:w281) -> (error out=w270:errorcluster, 3:w271:refnum<k16>)  [unwired: 1 in]
                    n197 = local read "IP_VS"() -> (w272:string)
                    n198 = local read "stateMachineCycle_uS"() -> (w351:i64)
                    n199 = local read "stateMachineCycle_uS"() -> (w330:i64)
                    n200 = String To IP(1:w272) -> (0:w273:u32)
                    n201 = UDP Write(address=w273, port or service name=u16 9093, connection ID=w271, data in="1", 8:w270) -> (error out=w268:errorcluster, 3:w269:refnum<k16>)  [unwired: 1 in]
                    n202 = local read "displayLength"() -> (w324:dbl)
                    n203 = local read "tickRate"() -> (w295:u32)
                    n204 = Divide(x=w351, y=sgl 50.0) -> (x/y=w350:sgl)
                    n205 = To Quad Integer(1:w350) -> (0:w304:i64)
                    n206 = Divide(x=w330, y=1000000.0) -> (x/y=w296:dbl)
                    n207 = Multiply(x=w296, y=w295) -> (x*y=w294:dbl)
                    n208 = Array Subset(array=w291, index=0, length=w297) -> (w341:sgl[])
                    n209 = Divide(x=w324, y=w294) -> (x/y=w327:dbl)
                    n210 = To Unsigned Long Integer(number=w327) -> (unsigned 32bit integer=w325:u32)
                    n211 = Initialize Array(u8 0, w325, 6 ("dimension size")) -> (w326:u8[][])
                    n212 = Initialize Array(u32 0, u32 4) -> (w288:u32[])
                    n213 = local read "trialKey"() -> (w267:i32[])
                    n214 = node-c288(w304) -> (w323:T4)  [unwired: 2 in]
                    n215 = node-c288(w304) -> (w321:T4)  [unwired: 2 in]
                    n216 = node-c288(w304) -> (w354:T4)  [unwired: 2 in]
                    n217 = node-c288(10) -> (w345:T4)  [unwired: 2 in]
                    n218 = timed-loop {
                      tunnel: w298 -> [w460]
                      tunnel: w299 -> [w459]
                      shift-right: [w431] -> _
                      shift-left: u32 0 -> [w448]
                      shift-right: [w454] -> _
                      shift-left: w326 -> [w456]
                      tunnel: w325 -> [w455]
                      timing: w323 -> [_]
                      timing-out: [_] -> w322
                      tunnel: [w451] -> w313
                      tunnel: [w450] -> w312
                      tunnel: w294 -> [w449]
                      shift-right: [w442] -> _
                      shift-left: w288 -> [w447]
                      stop <- w453 stop-if-true
                      n219 = node-c288() -> ()  [unwired: 1 in]
                      n220 = Dequeue Element(queue=w460, timeout in ms (-1)=0, error in (no error)=w459) -> (queue out=w451:refnum<queue>, element=w457:sgl[], timed out?=w458:bool, error out=w450:errorcluster)
                      n221 = case shown="False" w458 {
                        tunnel: w457 -> [w472 _]
                        tunnel: w448 -> [w471 w561]
                        tunnel: [w470 w561] -> w431
                        tunnel: w456 -> [w469 w562]
                        tunnel: w455 -> [w468 _]
                        tunnel: [w467 w562] -> w454
                        tunnel: [FALSE w563] -> w453
                        tunnel: w449 -> [w465 _]
                        tunnel: w447 -> [w464 w560]
                        tunnel: [w463 w560] -> w442
                        frame False {
                          n222 = stacked-sequence {
                            seq-local: [w474 _] -> [_ w531]
                            tunnel: w472 -> [w503 _]
                            tunnel: w471 -> [w488 _]
                            tunnel: [w493 _] -> w470
                            tunnel: w469 -> [_ w530]
                            tunnel: w468 -> [_ w522]
                            tunnel: [_ w525] -> w467
                            tunnel: w465 -> [_ w523]
                            tunnel: w464 -> [_ w505]
                            tunnel: [_ w504] -> w463
                            frame #0 {
                              w482 = sgl 9.0
                              # "display the last cycle in each stream"
                              # "find state 10:reward"
                              n223 = Decimate 1D Array(w503) -> (w489:sgl[], w491:sgl[], w490:sgl[], w474:sgl[])  [unwired: 5 out]
                              n224 = Array Size(array=w489) -> (size(s)=w487:i32)
                              n225 = Decrement(x=w487) -> (x-1=w486:i32)
                              n226 = Index Array(array=w489, index=w486) -> (element=w494:sgl)
                              n227 = Index Array(array=w491, index=w486) -> (element=→"CurTrial# (remote)":sgl)
                              n228 = Index Array(array=w490, index=w486) -> (element=w484:sgl)
                              "current state" <- w484
                              n229 = Array Subset(array=w490, index=0, length=w486) -> (w485:sgl[])
                              n230 = Divide(x=w494, y=sgl 1000000.0) -> (x/y=w496:sgl)
                              n231 = Quotient & Remainder(x=w496, y=sgl 60.0) -> (x-y*floor(x/y)=→"CurTime (sec)":sgl, floor(x/y)=→"CurTime":sgl)
                              n232 = feedback #1(sgl 0.0) -> (w499:sgl)
                              n233 = feedback-in #1(w484) -> ()
                              n234 = Build Array (concatenate)(w499, w485) -> (w483:sgl[])
                              n235 = Build Array (concatenate)(w485, w484) -> (w481:sgl[])
                              n236 = Equal?(x=w483, y=w482) -> (x = y?=w479:bool[])
                              n237 = Equal?(x=w482, y=w481) -> (x = y?=w478:bool[])
                              n238 = Boolean To (0,1)(Boolean=w478) -> (0, 1=w476:i16[])
                              n239 = Boolean To (0,1)(Boolean=w479) -> (0, 1=w477:i16[])
                              n240 = Less?(x=w477, y=w476) -> (x < y?=w480:bool[])
                              n241 = Boolean To (0,1)(Boolean=w480) -> (0, 1=w501:i16[])
                              n242 = Add Array Elements(numeric array=w501) -> (sum=w502:i16)
                              n243 = Add(x=w502, y=w488) -> (x+y=w493:u32)
                            }
                            frame #1 {
                              n244 = To Unsigned Word Integer(number=w531) -> (unsigned 16bit integer=w532:u16[])
                              n245 = for {
                                tunnel: w532 -> [w559] mode=indexing
                                tunnel: [w546] -> w514 mode=indexing
                                n246 = Number To Boolean Array(number=w559) -> (Boolean array=w558:bool[])
                                n247 = Index Array(array=w558, index #1=7, index #2=6, index #3=4, index #4=3, index #5=2, index #6=0) -> (element #1=w557:bool, element #2=w556:bool, element #3=w555:bool, element #4=w554:bool, element #5=w553:bool, element #6=w545:bool)
                                n248 = Build Array(w557, w556, w555, w554, w553, w545) -> (w547:bool[])
                                n249 = Boolean To (0,1)(Boolean=w547) -> (0, 1=w546:i16[])
                              }
                              n250 = Array Size(array=w531) -> (size(s)=w538:i32)
                              n251 = Negate(x=w538) -> (-x=w536:i32)
                              n252 = for {
                                N: 6 -> [_]
                                tunnel: w530 -> [w543]
                                tunnel: w536 -> [w540]
                                tunnel: [w539] -> w537 mode=indexing
                                i -> [w542]
                                n253 = Index Array(array=w543, index (col)=w542) -> (element=w541:u8[])  [unwired: 1 in]
                                n254 = Rotate 1D Array(1:w541, 2:w540) -> (0:w539:u8[])
                              }
                              n255 = Subtract(x=w522, y=w538) -> (x-y=w533:u32)
                              n256 = Transpose 2D Array(2D array=w537) -> (transposed array=w520:u8[][])
                              n257 = Array Size(array=w520) -> (size(s)=w521:i32[])
                              n258 = Replace Array Subset(array=w520, new element=w514, index (row)=w533, index (col)=0 ("disabled index (col)")) -> (w525:u8[][])
                              n259 = Index Array(array=w521) -> ()  [unwired: 1 in, 1 out]
                              n260 = Index Array(array=w514, index (col) #1=0, index (col) #2=1, index (col) #3=2, index (col) #4=3) -> (element #1=w515:i16[], element #2=w513:i16[], element #3=w512:i16[], element #4=w511:i16[])  [unwired: 4 in]
                              n261 = Bundle By Name ("Build Digital Data")("data"=w525) -> (w527:digitaldata)  [unwired: 1 in]
                              n262 = To Time Stamp(1:10.0 ("number")) -> (0:w529:timestamp)
                              n263 = Add Array Elements(numeric array=w515) -> (sum=w510:i16)
                              n264 = Add Array Elements(numeric array=w512) -> (sum=w509:i16)
                              n265 = Add Array Elements(numeric array=w513) -> (sum=w507:i16)
                              n266 = Add Array Elements(numeric array=w511) -> (sum=w508:i16)
                              n267 = call <vilib>:"DWDT Empty Digital.vi"() -> ("digital waveform out"=w526:digitalwaveform)  [unwired: 5 in]
                              n268 = Build Array(w510, w507, w509, w508) -> (w506:i16[])
                              n269 = Bundle By Name ("Build Waveform")(cluster=w526, "Y"=w527, "dt"=w523, "t0"=w529) -> (→"Digital Waveform Graph":digitalwaveform)
                              n270 = Add(x=w506, y=w505) -> (x+y=w504:u32[])
                            }
                          }
                        }
                        frame True {
                          n271 = local read "stop - local"() -> (w563:bool)
                        }
                      }
                      n272 = Index Array(array=w442, index #1=0, index #2=1, index #3=2, index #4=3) -> (element #1=w439:u32, element #2=w440:u32, element #3=w437:u32, element #4=w436:u32)
                      n273 = local write "reward#"(w448) -> ()
                      n274 = Add(x=w439, y=w440) -> (x+y=w441:u32)
                      n275 = Add(x=w437, y=w436) -> (x+y=w438:u32)
                      n276 = Divide(x=w439, y=w441) -> (x/y=w432:dbl)
                      n277 = Divide(x=w440, y=w441) -> (x/y=w433:dbl)
                      n278 = Divide(x=w437, y=w438) -> (x/y=w435:dbl)
                      n279 = Divide(x=w436, y=w438) -> (x/y=w434:dbl)
                      n280 = local write "rightReward"(w432) -> ()
                      n281 = local write "leftReward"(w433) -> ()
                      n282 = local write "rightLick"(w435) -> ()
                      n283 = local write "leftLick"(w434) -> ()
                      n284 = node-c288() -> ()  [unwired: 1 in, 1 out]
                    }
                    n285 = timed-loop {
                      timing: w321 -> [_]
                      timing-out: [_] -> w320
                      tunnel: w300 -> [w404]
                      tunnel: [w400] -> w319
                      shift-right: [w399] -> w318
                      shift-left: w301 -> [w403]
                      tunnel: w317 -> [w398]
                      tunnel: w316 -> [w397]
                      tunnel: [w396] -> w315
                      tunnel: [w395] -> w314
                      stop <- w394 stop-if-true
                      n286 = node-c288() -> ()  [unwired: 1 in, 1 out]
                      n287 = Dequeue Element(queue=w404, timeout in ms (-1)=0, error in (no error)=w403) -> (queue out=w400:refnum<queue>, element=w401:sgl[], timed out?=w402:bool, error out=w399:errorcluster)
                      n288 = case shown="False" w402 {
                        tunnel: w401 -> [w410 _]
                        tunnel: w398 -> [w409 w424]
                        tunnel: w397 -> [w408 w423]
                        tunnel: [w407 w424] -> w396
                        tunnel: [w406 w423] -> w395
                        tunnel: [_ w422] -> w394
                        frame False {
                          n289 = local read "Save data"() -> (w411:bool)
                          n290 = case shown="True" w411 {
                            tunnel: w409 -> [w412 w421]
                            tunnel: w408 -> [w413 w420]
                            tunnel: w410 -> [_ w415]
                            tunnel: [w413 w417] -> w406
                            tunnel: [w412 w416] -> w407
                            frame False {
                            }
                            frame True {
                              n291 = To Single Precision Float(number=w415) -> (single precision float=w414:sgl[])
                              n292 = Write to Binary File(file (use dialog)=w421, data=w414, error in=w420, 5:FALSE ("prepend array or string size? (T)"), 9:T3."little-endian" ("byte order (0:big-endian, network order)")) -> (refnum out=w416:refnum<file>, error out=w417:errorcluster)  [unwired: 1 in, 1 out]
                            }
                          }
                        }
                        frame True {
                          n293 = local read "stop - local"() -> (w422:bool)
                        }
                      }
                      n294 = node-c288() -> ()  [unwired: 1 in, 1 out]
                    }
                    n295 = timed-loop {
                      timing: w354 -> [_]
                      timing-out: [_] -> w353
                      tunnel: w304 -> [w1103]
                      tunnel: [w1121] -> w349
                      tunnel: w302 -> [w1120]
                      tunnel: w298 -> [w1119]
                      tunnel: w299 -> [w1118]
                      tunnel: w300 -> [w1117]
                      tunnel: w301 -> [w1116]
                      shift-right: [w1114] -> _
                      shift-left: w348 -> [w1115]
                      shift-right: [w1112] -> _
                      shift-left: w348 -> [w1113]
                      tunnel: [w1111] -> w306
                      tunnel: [w1110] -> w309
                      shift-right: [w1108] -> _
                      shift-left: u32 0 -> [w1109]
                      shift-right: [w1100] -> w346
                      shift-left: w303 -> [w1101]
                      stop <- w1097 stop-if-true
                      # "Ignore error stating the other\nendpoint has been destroyed."
                      n296 = node-c288() -> ()  [unwired: 1 in]
                      n297 = property class="Network Stream Endpoint"(reference=w1120, error in=w1101) -> (reference out=w1099:refnum<k21>, error out=w1104:errorcluster, "Connected"=w1124:bool, "AvailElmntsForRead"=w1125:i32)
                      n298 = local write "Available Elements for Writing"(w1125) -> ()
                      n299 = Not(x=w1124) -> (.not. x?=w1123:bool)
                      n300 = local write "Is Connected"(w1124) -> ()
                      n301 = shared-variable-read(w1099, w1104, w1103) -> (w1106:refnum<k21>, w1102:errorcluster, w1107:bool, w1105:sgl[])
                      n302 = Or(x=w1107, y=w1123) -> (x .or. y?=w1122:bool)
                      n303 = case shown="False" w1122 {
                        tunnel: w1106 -> [w1138 w1149]
                        tunnel: [w1138 w1149] -> w1121
                        tunnel: w1119 -> [w1142 _]
                        tunnel: w1118 -> [w1140 w1146]
                        tunnel: w1117 -> [w1141 _]
                        tunnel: w1116 -> [w1139 w1145]
                        tunnel: w1115 -> [w1136 w1148]
                        tunnel: [w1132 w1148] -> w1114
                        tunnel: w1113 -> [w1135 w1147]
                        tunnel: [w1134 w1147] -> w1112
                        tunnel: [w1131 w1146] -> w1111
                        tunnel: [w1130 w1145] -> w1110
                        tunnel: w1109 -> [w1129 w1144]
                        tunnel: [w1128 w1144] -> w1108
                        tunnel: w1105 -> [w1127 _]
                        tunnel: [w1126 w1143] -> w1098
                        tunnel: w1102 -> [w1126 w1143]
                        frame False {
                          n304 = Enqueue Element(queue=w1142, element=w1127, error in (no error)=w1140) -> (timed out?=w1137:bool, error out=w1131:errorcluster)  [unwired: 1 in, 1 out]
                          n305 = Enqueue Element(queue=w1141, element=w1127, error in (no error)=w1139) -> (timed out?=w1133:bool, error out=w1130:errorcluster)  [unwired: 1 in, 1 out]
                          n306 = Increment(x=w1129) -> (x+1=w1128:u32)
                          n307 = Or(x=w1137, y=w1136) -> (x .or. y?=w1132:bool)
                          n308 = Or(x=w1133, y=w1135) -> (x .or. y?=w1134:bool)
                          n309 = local write "stream counter"(w1128) -> ()
                          n310 = local write "saveTimeout"(w1134) -> ()
                          n311 = local write "dispTimeout"(w1132) -> ()
                        }
                        frame True {
                        }
                      }
                      n312 = shared-variable "Sabrina-RT1\\variables - network - RT (separate).lvlib\\stop - network"() -> (w1097:bool)  [unwired: 1 in, 1 out]
                      n313 = local write "stop - local"(w1097) -> ()
                      n314 = call "Remove_selected_error.vi"("error in (no error)"=w1098, "errorCode"=-314220) -> ("error out"=w1100:errorcluster)
                      n315 = node-c288() -> ()  [unwired: 1 in, 1 out]
                    }
                    n316 = timed-loop {
                      timing: w345 -> [_]
                      timing-out: [_] -> w344
                      tunnel: w343 -> [w605]
                      tunnel: w342 -> [w604]
                      shift-right: [w602] -> _
                      shift-left: w341 -> [w603]
                      tunnel: [w601] -> w340
                      tunnel: [w600] -> w339
                      shift-right: [w599] -> _
                      shift-left: 0 ("index") -> [w589]
                      shift-right: [w597] -> _
                      shift-left: FALSE -> [w598]
                      shift-right: [w595] -> w333
                      shift-left: w336 -> [w596]
                      tunnel: w269 -> [w593]
                      tunnel: w268 -> [w592]
                      tunnel: [w591] -> w283
                      tunnel: [w590] -> w282
                      shift-right: [w583] -> _
                      shift-left: w267 -> [w584]
                      stop <- w594 stop-if-true
                      n317 = node-c288() -> ()  [unwired: 1 in, 1 out]
                      n318 = local read "stateBusy"() -> (w608:bool)
                      n319 = local read "forceLeftTrial"() -> (w586:bool)
                      n320 = local read "forceRightTrial"() -> (w588:bool)
                      n321 = local read "VSbusy"() -> (w607:bool)
                      n322 = Exclusive Or(1:w588, 2:w586) -> (0:w587:bool)
                      n323 = case shown="False" w587 {
                        tunnel: w589 -> [_ w611]
                        tunnel: w586 -> [_ w613]
                        tunnel: [w609 w612] -> w585
                        tunnel: w584 -> [w609 w610]
                        frame False {
                        }
                        frame True {
                          n324 = Select(t=1 ("index"), s=w613, f=2 ("index")) -> (s? t:f=w616:i32)
                          n325 = Replace Array Subset(array=w610, new element=w616, index=w611) -> (w612:i32[])
                        }
                      }
                      n326 = Or(x=w608, y=w607) -> (x .or. y?=w606:bool)
                      n327 = case shown="False" w606 {
                        tunnel: w605 -> [w630 w895]
                        tunnel: w604 -> [w623 w894]
                        tunnel: w603 -> [w633 w893]
                        tunnel: [w622 w892] -> w602
                        tunnel: [w629 w891] -> w601
                        tunnel: [w624 w890] -> w600
                        tunnel: w589 -> [w620 w889]
                        tunnel: [w635 w888] -> w599
                        tunnel: w598 -> [w634 w885]
                        tunnel: [w621 w887] -> w597
                        tunnel: w596 -> [w632 w886]
                        tunnel: [w631 w886] -> w595
                        tunnel: [w619 w881] -> w591
                        tunnel: [w618 w882] -> w590
                        tunnel: w593 -> [w619 w884]
                        tunnel: w592 -> [w618 w883]
                        tunnel: w585 -> [w617 w880]
                        tunnel: [w617 w879] -> w583
                        frame False {
                          n328 = stacked-sequence {
                            seq-local: [_ w765 _] -> [_ _ w870]
                            tunnel: w620 -> [_ w760 w872]
                            tunnel: [_ _ w871] -> w635
                            tunnel: w634 -> [_ w804 _]
                            tunnel: w633 -> [_ w802 _]
                            tunnel: w632 -> [_ w762 _]
                            tunnel: [_ w796 _] -> w631
                            tunnel: [_ w794 _] -> w626
                            tunnel: [_ w770 _] -> w622
                            tunnel: [_ w765 _] -> w621
                            tunnel: w617 -> [_ w758 _]
                            frame #0 {
                              n329 = local read "No VS"() -> (w636:bool)
                              n330 = case shown="False" w636 {
                                frame True {
                                }
                                frame False {
                                n331 = local read "CurTrial#"() -> (w639:u16)
                                n332 = local read "autoTimeout"() -> (w649:bool)
                                n333 = case shown="True" w649 {
                                frame False {
                                }
                                frame True {
                                n334 = local read "curPerformance"() -> (w714:dbl)
                                n335 = local read "overallPerformance"() -> (w716:dbl)
                                n336 = local read "reward#"() -> (w717:i32)
                                n337 = Less?(x=w714, y=0.7) -> (x < y?=w719:bool)
                                n338 = Less?(x=w717, y=10 ("index")) -> (x < y?=w723:bool)
                                n339 = Less?(x=w716, y=0.3) -> (x < y?=w725:bool)
                                n340 = Or(x=w723, y=w725) -> (x .or. y?=w720:bool)
                                n341 = Not(x=w720) -> (.not. x?=w718:bool)
                                n342 = And(x=w718, y=w719) -> (x .and. y?=w721:bool)
                                n343 = case shown="True" w721 {
                                tunnel: [w729 w731] -> w722
                                frame False {
                                n344 = local read "timeout_uS"() -> (w729:u32)
                                }
                                frame True {
                                n345 = local read "CurTrial#"() -> (w730:u16)
                                n346 = Quotient & Remainder(x=w730, y="updateEveryTrial#") -> (x-y*floor(x/y)=w739:u16)  [unwired: 1 out]
                                n347 = Equal?(x=0.0, y=w739) -> (x = y?=w738:bool)
                                n348 = local read "timeout_uS"() -> (w735:u32)
                                n349 = Add(x=1000000, y=w735) -> (x+y=w736:u32)
                                n350 = Select(t=w736, s=w738, f=w735) -> (s? t:f=w733:u32)
                                n351 = Less?(x=w733, y="maxTimeout") -> (x < y?=w734:bool)
                                n352 = Select(t=w733, s=w734, f="maxTimeout") -> (s? t:f=w731:u32)
                                }
                                }
                                n353 = Select(t=0, s=w720, f=w722) -> (s? t:f=w727:u32)
                                n354 = local write "timeout_uS"(w727) -> ()
                                }
                                }
                                n355 = local read "reward#"() -> (w640:i32)
                                n356 = local read "autoCorrTrial"() -> (w650:bool)
                                n357 = Divide(x=w640, y=w639) -> (x/y=w638:dbl)
                                n358 = local write "overallPerformance"(w638) -> ()
                                n359 = case shown="True" w650 {
                                frame False {
                                }
                                frame True {
                                n360 = local read "overallPerformance"() -> (w742:dbl)
                                n361 = local read "rightReward"() -> (w751:dbl)
                                n362 = local read "leftReward"() -> (w743:dbl)
                                n363 = local read "reward#"() -> (w744:i32)
                                n364 = Greater Or Equal?(x=w744, y=10 ("index")) -> (x >= y?=w747:bool)
                                n365 = Max & Min(x=w751, y=w743) -> (max(x,y)=w755:dbl)  [unwired: 1 out]
                                n366 = Greater Or Equal?(x=w742, y=0.5) -> (x >= y?=w745:bool)
                                n367 = Less?(x=w755, y=0.55 ("number")) -> (x < y?=w748:bool)
                                n368 = And(x=w748, y=w745) -> (x .and. y?=w746:bool)
                                n369 = Select(t=FALSE, s=w746, f=w747) -> (s? t:f=w753:bool)
                                n370 = local write "forceCorrTrial"(w753) -> ()
                                }
                                }
                                n371 = local read "autoDelay"() -> (w637:bool)
                                n372 = case shown="True" w637 {
                                tunnel: [w651 w655] -> w641
                                frame False {
                                n373 = local read "overallPerformance"() -> (w651:dbl)
                                }
                                frame True {
                                n374 = local read "reward#"() -> (w652:i32)
                                n375 = Greater?(x=w652, y=u16 11) -> (0:w653:bool)
                                n376 = case shown="True" w653 {
                                tunnel: [w662 w670] -> w655
                                tunnel: w652 -> [w660 w663]
                                frame False {
                                n377 = Equal?(x=w660, y=u16 11) -> (x = y?=w659:bool)
                                n378 = local read "overallPerformance"() -> (w662:dbl)
                                n379 = Select(t="minDelay", s=w659, f=u32 0 ("delay_uS")) -> (s? t:f=w656:u32)
                                n380 = local write "delay_uS"(w656) -> ()
                                }
                                frame True {
                                n381 = local read "newStartReward#"() -> (w672:i32)
                                n382 = local read "newStartTrial#"() -> (w674:i32)
                                n383 = local read "contNoRewardAccum"() -> (w673:i32)
                                n384 = local read "CurTrial# (remote)"() -> (w664:u16)
                                n385 = Subtract(x=w663, y=w672) -> (x-y=w665:i32)
                                n386 = local read "contReward"() -> (w675:i32)
                                n387 = Subtract(x=w664, y=w674) -> (x-y=w668:i32)
                                n388 = Subtract(x=w668, y=w673) -> (x-y=w671:i32)
                                n389 = Less?(x=10 ("index"), y=w668) -> (x < y?=w667:bool)
                                n390 = Greater Or Equal?(x=w675, y=4) -> (x >= y?=w680:bool)
                                n391 = Divide(x=w665, y=w671) -> (x/y=w670:dbl)
                                n392 = Greater?(x=w663, y=14) -> (0:w679:bool)
                                n393 = And(x=w679, y=w680) -> (x .and. y?=w678:bool)
                                n394 = Greater?(x=w670, y=0.7 ("number")) -> (0:w666:bool)
                                n395 = Compound Arithmetic op=AND(w678, w667, w666) -> (w681:bool)
                                n396 = case shown="True" w681 {
                                tunnel: w664 -> [_ w688]
                                tunnel: w663 -> [_ w687]
                                frame False {
                                }
                                frame True {
                                w684 = 0
                                n397 = local read "delay_uS"() -> (w689:u32)
                                n398 = local write "newStartReward#"(w687) -> ()
                                n399 = local write "newStartTrial#"(w688) -> ()
                                n400 = Add(x=w689, y=200000.0 ("number")) -> (x+y=w683:dbl)
                                n401 = local write "contNoRewardAccum"(w684) -> ()
                                n402 = local write "contReward"(w684) -> ()
                                n403 = Max & Min(x="maxDelay", y=w683) -> (min(x,y)=w685:dbl)  [unwired: 1 out]
                                n404 = local write "delay_uS"(w685) -> ()
                                }
                                }
                                }
                                }
                                }
                                }
                                n405 = local read "autoAllowCorrection"() -> (w644:bool)
                                n406 = local read "contNoReward"() -> (w647:i32)
                                n407 = local read "autoStop"() -> (w648:bool)
                                n408 = case shown="True" w648 {
                                frame False {
                                }
                                frame True {
                                n409 = local read "overallPerformance"() -> (w704:dbl)
                                n410 = Multiply(x=0.9 ("y"), y="autoStopAtReward#") -> (x*y=w698:dbl)
                                n411 = Less?(x=w704, y=0.7) -> (x < y?=w701:bool)
                                n412 = local read "waterPunish"() -> (w702:bool)
                                n413 = And(x=w701, y=w702) -> (x .and. y?=w703:bool)
                                n414 = Select(t=w698, s=w703, f="autoStopAtReward#") -> (s? t:f=w708:dbl)
                                n415 = local read "contNoReward"() -> (w706:i32)
                                n416 = local read "reward#"() -> (w712:i32)
                                n417 = Greater Or Equal?(x=w712, y=w708) -> (x >= y?=w711:bool)
                                n418 = Greater?(x=w706, y=20 ("index")) -> (0:w705:bool)
                                n419 = Or(x=w711, y=w705) -> (x .or. y?=w710:bool)
                                n420 = case shown="True" w710 {
                                frame False {
                                }
                                frame True {
                                n421 = local write "run-stop"(FALSE) -> ()
                                }
                                }
                                }
                                }
                                n422 = Greater?(x=w647, y=5 ("index")) -> (0:w645:bool)
                                n423 = And(x=w645, y=w644) -> (x .and. y?=w643:bool)
                                n424 = case shown="False" w643 {
                                tunnel: [w691 TRUE] -> w642
                                frame False {
                                n425 = local read "reward#"() -> (w696:i32)
                                n426 = Greater Or Equal?(x=w696, y=10 ("index")) -> (x >= y?=w694:bool)
                                n427 = Select(t=FALSE, s=w694, f=TRUE) -> (s? t:f=w691:bool)
                                }
                                frame True {
                                }
                                }
                                n428 = local write "curPerformance"(w641) -> ()
                                n429 = local write "allowCorrection"(w642) -> ()
                                }
                              }
                            }
                            frame #1 {
                              # "beh para (20)"
                              n430 = local read "delay_uS"() -> (w792:u32)
                              n431 = local read "rewardPeriod_uS"() -> (w791:u32)
                              n432 = local read "rwdrefPeriod_uS"() -> (w790:u32)
                              n433 = local read "waterOn_uS"() -> (w789:u32)
                              n434 = local read "shockOn_uS"() -> (w788:u32)
                              n435 = local read "timeout_uS"() -> (w787:u32)
                              n436 = local read "lickReward"() -> (w786:bool)
                              n437 = local read "toneReward"() -> (w785:bool)
                              n438 = local read "allowPunish"() -> (w784:bool)
                              n439 = local read "manualShock"() -> (w783:bool)
                              n440 = local read "manualWaterLeft"() -> (w782:bool)
                              n441 = local read "manualWaterRight"() -> (w781:bool)
                              n442 = local read "lickThreshold_V"() -> (w780:fxp<+/-,16,5>)
                              n443 = local read "vsThreshold_V"() -> (w779:fxp<+/-,16,5>)
                              n444 = local read "audioThreshold_V"() -> (w778:fxp<+/-,16,5>)
                              n445 = local read "audioOffState_V"() -> (w775:fxp<+/-,16,5>)
                              n446 = local read "audioFilterPeriod_uS"() -> (w777:i32)
                              n447 = local read "vsFilterPeriod_uS"() -> (w776:i32)
                              n448 = local read "allowCorrection"() -> (w756:bool)
                              n449 = Index Array(array=w758, index=w760) -> (element=w761:i32)
                              n450 = Build Array(w792, w791, w790, w789, w788, w787) -> (w774:u32[])
                              n451 = Build Array(w786, w785, w784, w783, w782, w781, w756) -> (w767:bool[])
                              n452 = Boolean To (0,1)(Boolean=w767) -> (0, 1=w766:i16[])
                              n453 = Build Array(w780, w779, w778, w775, w777, w776) -> (w773:fxp<+/-,43,32>[])
                              n454 = Initialize Array(sgl 0.0, 1) -> (w757:sgl[])
                              n455 = Build Array (concatenate)(w774, w766, w773, w761, w757) -> (w770:sgl[])
                              n456 = Array Size(array=w770) -> (size(s)=w769:i32)
                              n457 = Subtract(x=w770, y=w802) -> (x-y=w801:sgl[])
                              n458 = Reshape Array(w770, w769, 1 ("dimension size")) -> (w797:sgl[][])
                              n459 = Absolute Value(x=w801) -> (abs(x)=w799:sgl[])
                              n460 = Less?(x=w799, y=1e-06) -> (x < y?=w798:bool[])
                              n461 = Replace Array Subset(array=w762, new element=w797, index (row)=0 ("dimension size"), index (col)=w760) -> (w796:sgl[][])
                              n462 = for {
                                N: 19 ("dimension size") -> [_]
                                tunnel: w798 -> [w841] mode=indexing
                                tunnel: w770 -> [w840] mode=indexing
                                shift-right: [w837] -> w795
                                shift-left: "" -> [w838]
                                i -> [w839]
                                n463 = case shown="False" w841 {
                                tunnel: w840 -> [_ w850]
                                tunnel: w839 -> [_ w844]
                                tunnel: w838 -> [w842 w848]
                                tunnel: [w842 w847] -> w837
                                frame True {
                                }
                                frame False {
                                n464 = case shown="3" w844 {
                                tunnel: ["dly" "rwp" "rwf" "wdr" "shd" "tod" "lkr" "tlr" "alp" "msh" "mwl" "mwr" "alc" "lth" "vth" "ath" "aof" "afp" _ _ _] -> w843
                                frame 0, Default {
                                }
                                frame 1 {
                                }
                                frame 2 {
                                }
                                frame 3 {
                                }
                                frame 4 {
                                }
                                frame 5 {
                                }
                                frame 6 {
                                }
                                frame 7 {
                                }
                                frame 8 {
                                }
                                frame 9 {
                                }
                                frame 10 {
                                }
                                frame 11 {
                                }
                                frame 12 {
                                }
                                frame 13 {
                                }
                                frame 14 {
                                }
                                frame 15 {
                                }
                                frame 16 {
                                }
                                frame 17 {
                                }
                                frame 18 {
                                (unwired) "vfp"
                                }
                                frame 19 {
                                }
                                frame 20 {
                                }
                                }
                                n465 = Format Value(format string="%.3f", value (0)=w850) -> (output string=w845:string)  [unwired: 1 in]
                                n466 = call <vilib>:"Space Constant.vi"() -> ("String"=w846:string)
                                n467 = Concatenate Strings(w848, w843, w846, w845, w846) -> (w847:string)
                                }
                                }
                              }
                              n468 = local read "VSmissed"() -> (w807:bool)
                              n469 = local read "stateMissed"() -> (w806:bool)
                              n470 = local read "CurTrial#"() -> (w810:u16)
                              n471 = local read "totalTrial#"() -> (w809:u16)
                              n472 = local read "run-stop"() -> (w805:bool)
                              n473 = Equal?(x=w810, y=w809) -> (x = y?=w808:bool)
                              n474 = Not(x=w805) -> (.not. x?=w803:bool)
                              n475 = Compound Arithmetic op=OR(w807, w806, w808) -> (w793:bool)
                              n476 = case shown="True" w793 {
                                frame False {
                                }
                                frame True {
                                n477 = local write "run-stop"(FALSE ("run-stop")) -> ()
                                }
                              }
                              n478 = Compound Arithmetic op=OR(w793, w803, w804) -> (w765:bool)
                              n479 = case shown="True" w765 {
                                tunnel: w795 -> [w814 _]
                                tunnel: [w813 w833] -> w794
                                tunnel: w761 -> [w811 _]
                                frame False {
                                n480 = flat-sequence {
                                tunnel: w814 -> [w815]
                                tunnel: [w815] -> w812
                                tunnel: [w829] -> w813
                                tunnel: w812 -> [w832]
                                tunnel: w811 -> [w826]
                                frame #0 {
                                n481 = disable-structure shown="Enabled" {
                                frame Disabled {
                                n482 = Random Number (0-1)() -> (number: 0 to 1=w818:dbl)
                                n483 = Multiply(x=w818, y=3000.0) -> (x*y=w820:dbl)
                                n484 = local read "ITI_ms"() -> (w816:dbl)
                                n485 = Add(x=w816, y=w820) -> (x+y=w819:dbl)
                                n486 = Wait (ms)(milliseconds to wait=w819) -> ()  [unwired: 1 out]
                                }
                                frame Enabled {
                                n487 = Random Number (0-1)() -> (number: 0 to 1=w823:dbl)
                                n488 = local read "ITI_ms"() -> (w821:dbl)
                                n489 = Multiply(x=w823, y=0) -> (x*y=w822:dbl)
                                n490 = Add(x=w821, y=w822) -> (x+y=w824:dbl)
                                n491 = Wait (ms)(milliseconds to wait=w824) -> ()  [unwired: 1 out]
                                }
                                }
                                }
                                frame #1 {
                                n492 = call <vilib>:"Space Constant.vi"() -> ("String"=w830:string)
                                n493 = Format Value(format string="%.3f", value (0)=w826) -> (output string=w827:string)  [unwired: 1 in]
                                n494 = Concatenate Strings(w832, "start" ("string"), w830, w827, w830) -> (w829:string)
                                }
                                }
                                }
                                frame True {
                                n495 = call <vilib>:"Space Constant.vi"() -> ("String"=w835:string)
                                n496 = Concatenate Strings("stop" ("string"), w835, "1.000" ("string"), w835) -> (w833:string)
                                n497 = call "generateTone.vi"() -> ()  [unwired: 12 in]
                                }
                              }
                            }
                            frame #2 {
                              n498 = case shown="False" w870 {
                                tunnel: w872 -> [w873 w878]
                                tunnel: [w873 w877] -> w871
                                frame True {
                                }
                                frame False {
                                n499 = Increment(x=w878) -> (x+1=w877:i32)
                                n500 = local read "No VS"() -> (w874:bool)
                                n501 = Not(x=w874) -> (.not. x?=w875:bool)
                                n502 = local write "CurTrial#"(w877) -> ()
                                n503 = local write "stateBusy"(TRUE) -> ()
                                n504 = local write "VSbusy"(w875) -> ()
                                }
                              }
                            }
                          }
                          n505 = local write "INFO"(w626) -> ()
                          n506 = local read "IP_broadcast"() -> (w627:string)
                          n507 = local read "port_remote"() -> (w625:u16)
                          n508 = String To IP(1:w627) -> (0:w628:u32)
                          n509 = UDP Write(address=w628, port or service name=w625, connection ID=w630, data in=w626, 8:w623) -> (error out=w624:errorcluster, 3:w629:refnum<k16>)  [unwired: 1 in]
                        }
                        frame True {
                          n510 = stacked-sequence {
                            tunnel: w895 -> [w949 _]
                            tunnel: w894 -> [w948 _]
                            tunnel: w893 -> [w944 _]
                            tunnel: [w907 _] -> w892
                            tunnel: [w902 _] -> w891
                            tunnel: [w903 _] -> w890
                            tunnel: w889 -> [w900 w1002]
                            tunnel: [_ w1001] -> w888
                            tunnel: [w930 _] -> w887
                            tunnel: w885 -> [w904 _]
                            tunnel: w884 -> [_ w1000]
                            tunnel: w883 -> [_ w999]
                            tunnel: [_ w998] -> w881
                            tunnel: [_ w997] -> w882
                            tunnel: w880 -> [w897 w995]
                            tunnel: [_ w994] -> w879
                            frame #0 {
                              # "triakKey is not used here, may be deleted"
                              # "beh para (21)"
                              n511 = local read "delay_uS"() -> (w929:u32)
                              n512 = local read "rewardPeriod_uS"() -> (w928:u32)
                              n513 = local read "rwdrefPeriod_uS"() -> (w927:u32)
                              n514 = local read "waterOn_uS"() -> (w926:u32)
                              n515 = local read "shockOn_uS"() -> (w925:u32)
                              n516 = local read "timeout_uS"() -> (w924:u32)
                              n517 = local read "lickReward"() -> (w923:bool)
                              n518 = local read "toneReward"() -> (w922:bool)
                              n519 = local read "allowPunish"() -> (w921:bool)
                              n520 = local read "manualShock"() -> (w920:bool)
                              n521 = local read "manualWaterLeft"() -> (w919:bool)
                              n522 = local read "manualWaterRight"() -> (w918:bool)
                              n523 = local read "lickThreshold_V"() -> (w917:fxp<+/-,16,5>)
                              n524 = local read "vsThreshold_V"() -> (w916:fxp<+/-,16,5>)
                              n525 = local read "audioThreshold_V"() -> (w915:fxp<+/-,16,5>)
                              n526 = local read "audioOffState_V"() -> (w912:fxp<+/-,16,5>)
                              n527 = local read "audioFilterPeriod_uS"() -> (w914:i32)
                              n528 = local read "vsFilterPeriod_uS"() -> (w913:i32)
                              n529 = local read "allowCorrection"() -> (w896:bool)
                              n530 = Index Array(array=w897, index=w900) -> (element=w899:i32)
                              n531 = Build Array(w929, w928, w927, w926, w925, w924) -> (w911:u32[])
                              n532 = Build Array(w923, w922, w921, w920, w919, w918, w896) -> (w906:bool[])
                              n533 = Boolean To (0,1)(Boolean=w906) -> (0, 1=w905:i16[])
                              n534 = Build Array(w917, w916, w915, w912, w914, w913) -> (w910:fxp<+/-,43,32>[])
                              n535 = Initialize Array(sgl 0.0, 1) -> (w901:sgl[])
                              n536 = Build Array (concatenate)(w911, w905, w910, w899, w901) -> (w907:sgl[])
                              n537 = Subtract(x=w907, y=w944) -> (x-y=w947:sgl[])
                              n538 = Absolute Value(x=w947) -> (abs(x)=w946:sgl[])
                              n539 = Less?(x=w946, y=1e-06) -> (x < y?=w943:bool[])
                              n540 = for {
                                N: 19 ("dimension size") -> [_]
                                tunnel: w943 -> [w952] mode=indexing
                                shift-right: [w953] -> w939
                                shift-left: "" -> [w954]
                                tunnel: w907 -> [w951] mode=indexing
                                i -> [w955]
                                n541 = case shown="False" w952 {
                                tunnel: w955 -> [w963 _]
                                tunnel: w954 -> [w959 w983]
                                tunnel: [w957 w983] -> w953
                                tunnel: w951 -> [w956 _]
                                frame False {
                                n542 = case shown="15" w963 {
                                tunnel: ["dly" "rwp" "rwf" "wdr" "shd" "tod" "lkr" "tlr" "alp" "msh" "mwl" "mwr" "alc" "lth" "vth" "ath" "aof" "afp" "vfp" _ _] -> w958
                                frame 0, Default {
                                }
                                frame 1 {
                                }
                                frame 2 {
                                }
                                frame 3 {
                                }
                                frame 4 {
                                }
                                frame 5 {
                                }
                                frame 6 {
                                }
                                frame 7 {
                                }
                                frame 8 {
                                }
                                frame 9 {
                                }
                                frame 10 {
                                }
                                frame 11 {
                                }
                                frame 12 {
                                }
                                frame 13 {
                                }
                                frame 14 {
                                }
                                frame 15 {
                                }
                                frame 16 {
                                }
                                frame 17 {
                                }
                                frame 18 {
                                }
                                frame 19 {
                                }
                                frame 20 {
                                }
                                }
                                n543 = Format Value(format string="%.3f", value (0)=w956) -> (output string=w960:string)  [unwired: 1 in]
                                n544 = call <vilib>:"Space Constant.vi"() -> ("String"=w961:string)
                                n545 = Concatenate Strings(w959, w958, w961, w960, w961) -> (w957:string)
                                }
                                frame True {
                                }
                                }
                              }
                              n546 = String Length(string=w939) -> (length=w940:i32)
                              n547 = Not Equal To 0?(x=w940) -> (x != 0?=w941:bool)
                              n548 = case shown="True" w941 {
                                tunnel: w949 -> [w984 w993]
                                tunnel: w948 -> [w985 w992]
                                tunnel: w939 -> [_ w988]
                                tunnel: [w984 w987] -> w902
                                tunnel: [w985 w986] -> w903
                                frame False {
                                }
                                frame True {
                                n549 = local read "IP_broadcast"() -> (w990:string)
                                n550 = local read "port_remote"() -> (w989:u16)
                                n551 = String To IP(1:w990) -> (0:w991:u32)
                                n552 = UDP Write(address=w991, port or service name=w989, connection ID=w993, data in=w988, 8:w992) -> (error out=w986:errorcluster, 3:w987:refnum<k16>)  [unwired: 1 in]
                                }
                              }
                              n553 = local read "VSmissed"() -> (w934:bool)
                              n554 = local read "stateMissed"() -> (w935:bool)
                              n555 = local read "CurTrial#"() -> (w931:u16)
                              n556 = local read "totalTrial#"() -> (w932:u16)
                              n557 = local read "run-stop"() -> (w938:bool)
                              n558 = Equal?(x=w931, y=w932) -> (x = y?=w933:bool)
                              n559 = Not(x=w938) -> (.not. x?=w937:bool)
                              n560 = Compound Arithmetic op=OR(w934, w935, w933) -> (w936:bool)
                              n561 = case shown="False" w936 {
                                frame False {
                                }
                                frame True {
                                n562 = local write "run-stop"(FALSE ("run-stop")) -> ()
                                }
                              }
                              n563 = Compound Arithmetic op=OR(w936, w937, w904) -> (w930:bool)
                            }
                            frame #1 {
                              n564 = UDP Read(connection ID=w1000, timeout ms (25000)=0, 8:w999) -> (data out=w1003:string, error out=w1008:errorcluster, 3:w998:refnum<k16>, 6:w1004:u32)  [unwired: 1 in, 1 out]
                              n565 = String Length(string=w1003) -> (length=w1006:i32)
                              n566 = local write "Incoming data"(w1003) -> ()
                              n567 = Not Equal To 0?(x=w1006) -> (x != 0?=w1005:bool)
                              n568 = case shown="True" w1005 {
                                tunnel: w1004 -> [_ w1016]
                                tunnel: w1003 -> [_ w1022]
                                tunnel: w1002 -> [w1010 w1015]
                                tunnel: [w1010 w1013] -> w1001
                                tunnel: w995 -> [w1009 w1012]
                                tunnel: [w1009 w1011] -> w994
                                frame False {
                                }
                                frame True {
                                n569 = Scan From String(format string="%s %f ", input string=w1022, initial scan location=u32 0, default 1="no" ("default value 1"), default 2=-1.0 ("default value 2")) -> (output 1=w1017:string, output 2=w1014:dbl)  [unwired: 1 in, 3 out]
                                n570 = case shown="\"TrlDone\", Default" w1017 {
                                tunnel: w1016 -> [w1032]
                                tunnel: w1015 -> [w1025]
                                tunnel: w1014 -> [w1026]
                                tunnel: [w1025] -> w1013
                                tunnel: w1012 -> [w1024]
                                tunnel: [w1023] -> w1011
                                frame "TrlDone", Default {
                                n571 = local read "IP_RT"() -> (w1030:string)
                                n572 = IP To String(1:TRUE ("dot notation? (F)"), 2:w1032) -> (0:w1027:string)
                                n573 = Match True/False String(2:"" ("false string"), 3:w1030, 4:w1027) -> (0:w1028:bool)  [unwired: 1 out]
                                n574 = local write "Originating IP"(w1027) -> ()
                                n575 = case shown="False" w1028 {
                                tunnel: w1027 -> [w1039 _]
                                tunnel: w1025 -> [w1036 w1057]
                                tunnel: w1026 -> [w1035 w1051]
                                tunnel: w1024 -> [w1033 w1056]
                                tunnel: [w1033 w1055] -> w1023
                                frame False {
                                n576 = local read "IP_VS"() -> (w1038:string)
                                n577 = Match True/False String(2:"" ("false string"), 3:w1038, 4:w1039) -> (0:w1034:bool)  [unwired: 1 out]
                                n578 = case shown="True" w1034 {
                                tunnel: w1036 -> [_ w1046]
                                tunnel: w1035 -> [_ w1045]
                                frame False {
                                n579 = local write "Error 2"("Unknown source Error") -> ()
                                }
                                frame True {
                                n580 = Subtract(x=w1045, y=w1046) -> (x-y=w1044:dbl)
                                n581 = Absolute Value(x=w1044) -> (abs(x)=w1043:dbl)
                                n582 = local write "VSbusy"(FALSE) -> ()
                                n583 = Greater?(x=w1043, y=1e-06) -> (0:w1041:bool)
                                n584 = local write "VSmissed"(w1041) -> ()
                                }
                                }
                                }
                                frame True {
                                n585 = To Word Integer(number=w1051) -> (16bit integer=w1054:i16)
                                n586 = local read "forceCorrTrial"() -> (w1053:bool)
                                n587 = To Word Integer(number=w1051) -> (16bit integer=w1050:i16)
                                n588 = disable-structure shown="Disabled" {
                                disable-tunnel: w1051 -> [w1089 _]
                                disable-tunnel: w1057 -> [w1088 _]
                                frame Disabled {
                                n589 = Subtract(x=w1089, y=w1088) -> (x-y=w1087:dbl)
                                n590 = Absolute Value(x=w1087) -> (abs(x)=w1086:dbl)
                                n591 = Greater?(x=w1086, y=1e-06) -> (0:w1084:bool)
                                n592 = local write "stateMissed"(w1084) -> ()
                                }
                                frame Enabled {
                                }
                                }
                                n593 = local write "stateBusy"(FALSE) -> ()
                                n594 = case shown="0, Default" w1050 {
                                tunnel: [w1061 0] -> w1052
                                tunnel: [0 w1071] -> w1049
                                tunnel: [w1059 w1063] -> w1048
                                frame 0, Default {
                                n595 = local read "contNoRewardAccum"() -> (w1059:i32)
                                n596 = local read "contNoReward"() -> (w1062:i32)
                                n597 = Increment(x=w1062) -> (x+1=w1061:i32)
                                }
                                frame 1 {
                                n598 = local read "contNoReward"() -> (w1067:i32)
                                n599 = Greater?(x=w1067, y=5) -> (0:w1068:bool)
                                n600 = Select(t=w1067, s=w1068, f=0) -> (s? t:f=w1066:i32)
                                n601 = local read "contNoRewardAccum"() -> (w1065:i32)
                                n602 = local read "contReward"() -> (w1070:i32)
                                n603 = Add(x=w1066, y=w1065) -> (x+y=w1063:i32)
                                n604 = Increment(x=w1070) -> (x+1=w1071:i32)
                                }
                                }
                                n605 = case shown="True" w1053 {
                                tunnel: w1057 -> [_ w1077]
                                tunnel: w1056 -> [w1073 w1076]
                                tunnel: [w1073 w1075] -> w1055
                                tunnel: w1054 -> [_ w1074]
                                frame False {
                                }
                                frame True {
                                n606 = case shown="0" w1074 {
                                tunnel: w1077 -> [w1079 _]
                                tunnel: w1076 -> [w1082 w1083]
                                tunnel: [w1080 w1083] -> w1075
                                frame 0 {
                                n607 = Decrement(x=w1079) -> (x-1=w1078:i32)
                                n608 = Index Array(array=w1082, index=w1078) -> (element=w1081:i32)
                                n609 = Replace Array Subset(array=w1082, new element=w1081, index=w1079) -> (w1080:i32[])
                                }
                                frame 1, Default {
                                }
                                }
                                }
                                }
                                n610 = local write "contNoReward"(w1052) -> ()
                                n611 = local write "contReward"(w1049) -> ()
                                n612 = local write "contNoRewardAccum"(w1048) -> ()
                                }
                                }
                                }
                                }
                                }
                              }
                              n613 = call "Remove_selected_error.vi"("error in (no error)"=w1008, "errorCode"=56) -> ("error out"=w997:errorcluster)
                            }
                          }
                        }
                      }
                      n614 = local read "stop - local"() -> (w594:bool)
                      n615 = node-c288() -> ()  [unwired: 1 in, 1 out]
                    }
                    n616 = node-c288(w320) -> ()  [unwired: 1 out]
                    n617 = Release Queue(queue=w319, error in (no error)=w318) -> (error out=w308:errorcluster)  [unwired: 1 in, 2 out]
                    n618 = To Single Precision Float(number=w333) -> (single precision float=w335:sgl[][])
                    n619 = local read "Save data"() -> (w334:bool)
                    n620 = node-c288(w353) -> ()  [unwired: 1 out]
                    n621 = case shown="True" w334 {
                      tunnel: w314 -> [w568 w582]
                      tunnel: w315 -> [_ w581]
                      tunnel: w335 -> [_ w572]
                      tunnel: [w568 w569] -> w307
                      frame False {
                      }
                      frame True {
                        n622 = Multiply(x=502, y=4) -> (x*y=w577:i32)
                        n623 = Set File Position(offset (in bytes) (0)=w577, refnum=w581, from (0:start)=enum16{"start", "end", "current"}."start", error in=w582) -> (refnum out=w574:refnum<file>, error out=w575:errorcluster)
                        n624 = Write to Binary File(file (use dialog)=w574, data=w572, error in=w575, 5:FALSE ("prepend array or string size? (T)"), 9:T3."little-endian" ("byte order (0:big-endian, network order)")) -> (refnum out=w570:refnum<file>, error out=w571:errorcluster)  [unwired: 1 in, 1 out]
                        n625 = Close File(refnum=w570, error in=w571) -> (error out=w569:errorcluster)  [unwired: 1 out]
                      }
                    }
                    n626 = node-c288(w322) -> ()  [unwired: 1 out]
                    n627 = Release Queue(queue=w313, error in (no error)=w312) -> (error out=w287:errorcluster)  [unwired: 1 in, 2 out]
                    n628 = Destroy Stream Endpoint(8:w346, 11:w349) -> (0:w310:errorcluster)
                    n629 = node-c288(w344) -> ()  [unwired: 1 out]
                    n630 = flat-sequence {
                      tunnel: w305 -> [w392]
                      frame #0 {
                        n631 = call <vilib>:"Simple Error Handler.vi"("error in (no error)"=w392) -> ()  [unwired: 4 in, 5 out]
                        n632 = shared-variable "Sabrina-RT1\\variables - network - RT (separate).lvlib\\stop - network"(FALSE ("stop - network")) -> ()  [unwired: 1 in, 1 out]
                      }
                    }
                    n633 = UDP Close(connection ID=w283, 8:w282) -> ()  [unwired: 2 out]
                    n634 = UDP Close(connection ID=w340, 8:w339) -> (error out=w311:errorcluster)  [unwired: 1 out]
                    n635 = Merge Errors(w311, w310, w306, w309, w287, w308, w307) -> (w305:errorcluster)
                  }
                }
              }
              frame 2 {
                n636 = local read "IP_host"() -> (w1160:string)
                n637 = local read "port_local"() -> (w1161:u16)
                n638 = String To IP(1:w1160) -> (0:w1159:u32)
                n639 = UDP Open(7:w1159, 11:w1161) -> (port=w1163:refnum<k16>, 0:w1164:errorcluster)  [unwired: 3 in, 1 out]
                n640 = local read "IP_broadcast"() -> (w1157:string)
                n641 = local read "port_remote"() -> (w1158:u16)
                n642 = String To IP(1:w1157) -> (0:w1162:u32)
                n643 = UDP Write(address=w1162, port or service name=w1158, connection ID=w1163, data in="exit 1.000 ", 8:w1164) -> (error out=w1166:errorcluster, 3:w1165:refnum<k16>)  [unwired: 1 in]
                n644 = UDP Close(connection ID=w1165, 8:w1166) -> (error out=w1167:errorcluster)  [unwired: 1 out]
                n645 = call <vilib>:"Simple Error Handler.vi"("error in (no error)"=w1167) -> ()  [unwired: 4 in, 5 out]
              }
            }
          }
          frame #2 {
            n646 = Wait (ms)(milliseconds to wait=u32 5) -> ()  [unwired: 1 out]
          }
        }
      }
    }
  }
